vi "GUI_Tape_Alignment.vi"() -> ()   [LabVIEW 2020]
uses:
  Shared/GUI_Template/GUI_master/tcp_new_data_event.ctl
  Shared/GUI_Template/GUI_master/tcp new data cluster.ctl
  <vilib>/addons/_JKI.lib/Network_Streams_Connection.llb/NetworkCommand--Cluster.ctl
  <vilib>/addons/_JKI.lib/Network_Streams_Connection.llb/PublicSettings.ctl
  <vilib>/addons/_JKI.lib/Network_Streams_Connection.llb/NetworkConnection.lvclass/NetworkConnection.ctl
  <vilib>/Analysis/NI_AALPro.lvlib
  <vilib>/addons/_JKI.lib/Network_Streams_Connection.llb/NetworkConnection.lvclass
panel:
  in  "Check beam quality":bool
  in  "Zpos Scan":bool
  in  "2ndmomW0y::1":dbl caption="w0 Y" min=0.0 max=999999.0
  in  "MaxCounts::1":dbl caption="Max Counts" min=0.0 max=999999999.0
  in  "xyzuvw::2":string caption="Hex position"
  out "slow response":string
  in  "?":T1(tab)
  out "Zpos and w0 Y":dbl(graph)
  out "Alignment attempts":i32
  out "Waveform Chart 2":u32(graph)
  out "Movement time":u32
  out "Alignment time":u32
  out "Waveform Chart 3":u32(graph)
  out "Waveform Chart 4":i32(graph)
  out "Waveform Chart":cluster{"centroidx::1":dbl, "centroidy::1":dbl}(graph)
  out "Zpos and w0 Y 2":dbl(graph)
  out "X Graph":T2(graph)
  out "Y Graph":T3(graph)
  out "X slope":dbl
  out "Y slope":dbl
  out "Y error":dbl
  out "X error":dbl
  in  "Calibration steps":dbl=8.0
  in  "Calibration Angle":cluster{"X":dbl, "Y":dbl}={"X"=0.01, "Y"=0.01}
  in  "Export":bool caption="Export calibration"
  in  "Import":bool caption="Import calibration"
  in  "Diagnostic type":enum16{"Max counts", "w0 Y"}(ring)
  in  "Disable Zpos Scan":bool
  in  "zpos scan increment":dbl=0.1
  in  "zpos scan range":dbl=2.0
  in  "w0 Y Cutoff":dbl=60.0
  in  "Buffer":dbl=0.9 format="%#_13g"
  in  "Accuracy limit":cluster{"X":dbl, "Y":dbl}={"X"=5.0, "Y"=5.0}
  in  "Disable pointing correction":bool
  in  "Max counts cutoff":dbl=2000.0
  out "Connected?":bool
  in  "Message To Send":T4={"Command"="Alignment Done!", "Arguments"=variant(string "Arguments are variants. Wire anything!"), " Msg Id"=0}
  in  "Settings":T5={"My Name"="AlignmentGUI", "Remote IP Address"="", "Remote Name"="TapeDrive"}
  out "Public Settings":T5
  out "Message count":i32
  out "Incoming Messages":T4[](array[typedef])
  in  "Target.Y::1":dbl caption="Target Y" min=0.0 max=2000.0
  in  "Target.X::1":dbl caption="Target X" min=0.0 max=2000.0
  in  "Stop":bool
  out "Remaining States":string
  out "Current State":string
  in  "Calibrate":bool
  in  "wangle::2":dbl caption="W" min=-10.0 max=10.0 step=0.01 format="%.5f"
  in  "vangle::2":dbl caption="V" min=-5.0 max=5.0 step=0.01 format="%.5f"
  in  "centroidy::1":dbl caption="Centroid Y" min=0.0 max=0.0
  in  "centroidx::1":dbl caption="Centroid X" min=0.0 max=0.0
  in  "ypos::2":dbl caption="Y" min=-25.0 max=25.0 step=0.01 format="%.5f"
  in  "xpos::2":dbl caption="X" min=-25.0 max=25.0 step=0.01 format="%.5f"
  in  "zpos::2":dbl caption="Z" min=-25.0 max=25.0 step=0.01 format="%.5f"
  in  "uangle::2":dbl caption="U" min=-5.0 max=5.0 step=0.01 format="%.5f"
  out "tcp data event":T6
  out "error IO 2":errorcluster
  in  "GUIdevice 2":string="HEX-PL1-2"
  in  "GUIdevice 1":string="CAM-PL1-SideSpec"
  in  "Align Tape":bool
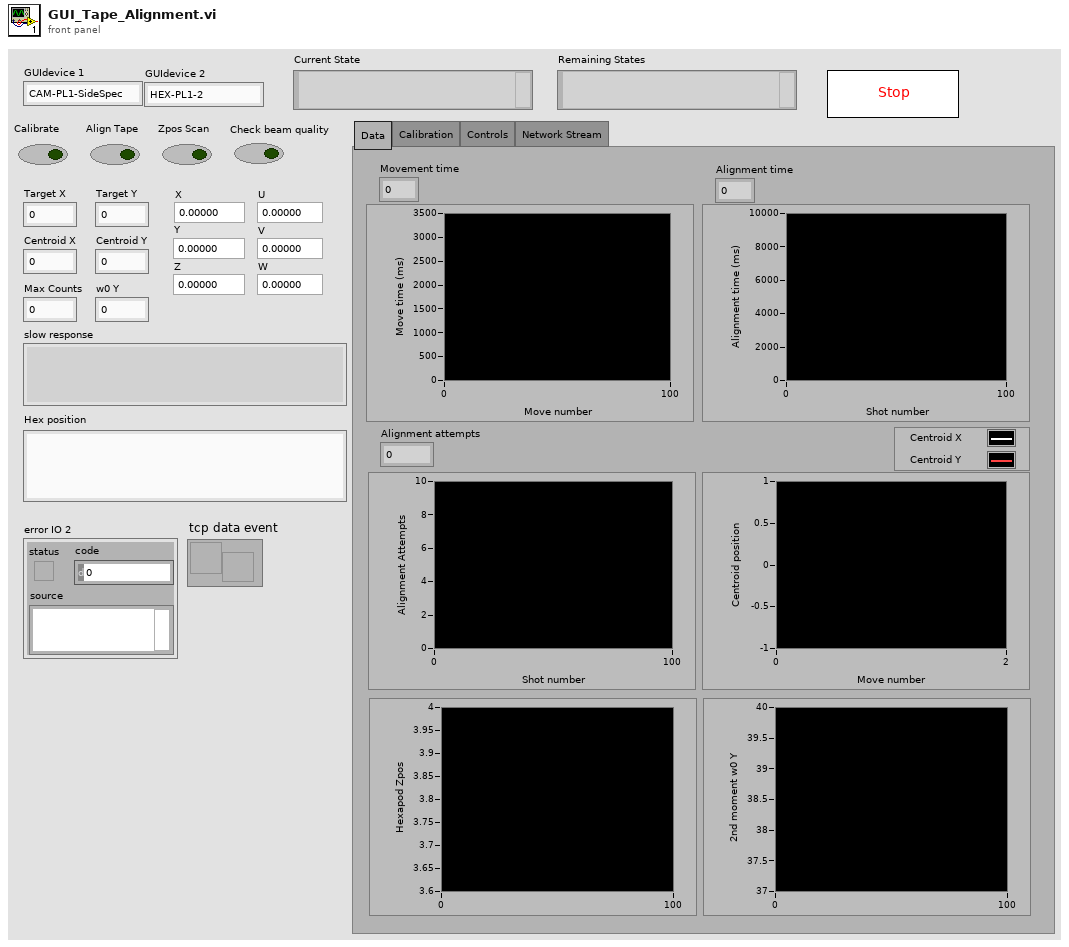
[diagram p1: front panel]
types:
  T1 = enum32{"Data", "Calibration", "Controls", "Network Stream"}
  T2 = cluster{"Centroids.x":dbl[], "Best Linear Fit":dbl[]}[]
  T3 = cluster{"Centroids.y":dbl[], "Best Linear Fit":dbl[]}[]
  T4 = typedef "NetworkConnection.lvclass/NetworkCommand--Cluster.ctl" = cluster{"Command":string, "Arguments":variant, " Msg Id":i32}
  T5 = typedef "NetworkConnection.lvclass/PublicSettings.ctl" = cluster{"My Name":string, "Remote IP Address":string, "Remote Name":string}
  T6 = typedef "tcp_new_data_event.ctl" = refnum<user-event>
  T7 = typedef "tcp new data cluster.ctl" = cluster{"EventEnum":enum16{"new data", "connection status update"}, "Device name":string}
  T8 = enum32{"Invalid", "Standard", "Closed", "Hidden", "Minimized", "Maximized"}
  T9 = enum32{"invalid app kind", "Development System", "Run Time System", "Student Edition", "Embedded LabVIEW", "Evaluation", "Custom"}
  T10 = cluster{"Messages[0]":T4, "Messages[1]":T4, "Messages[2]":T4, "Messages[3]":T4, "Messages[4]":T4, "Messages[5]":T4, "Messages[6]":T4, "Messages[7]":T4, "Messages[8]":T4}
  T11 = cluster{"Core":cluster{"Current VI Reference":refnum<vi>, "Close Panel on Exit?":bool}, "Difference":cluster{"X":dbl, "Y":dbl}, "Scale Factor":cluster{"X":dbl, "Y":dbl}, "Centroids":cluster{"Centroids.x":dbl[], "Centroids.y":dbl[]}, "Calibration Angle ":cluster{"X":dbl, "Y":dbl}, "Accuracy limit":cluster{"X":dbl, "Y":dbl}, "Calibration steps":dbl, "NetworkConnection out":refnum<class "NetworkConnection.lvclass">, "Messages":i32, "Alignment attempts":i32, "Timer":cluster{"T1":i32, "T2":i32}, "Hexapod positions":cluster{"P1":string, "P2":string}, "Beam diagnostic cutoffs":cluster{"MaxCounts":dbl, "w0 Y":dbl}, "Hexapod zscan data":cluster{"Hexapod zscan positions":dbl[], "Hexapod zscan diagnostic":dbl[], "Index":i32, "Best Zpos":dbl}, "Diagnostic type":string}
  T12 = cluster{"Hexapod zscan positions":dbl[], "Hexapod zscan diagnostic":dbl[], "Index":i32, "Best Zpos":dbl}
  T13 = cluster{"Centroids.x":dbl[], "Centroids.y":dbl[]}
  T14 = cluster{"Current VI Reference":refnum<vi>, "Close Panel on Exit?":bool}
  T15 = cluster{"Centroids.x":dbl[], "Best Linear Fit":dbl[]}
  T16 = cluster{"Centroids.y":dbl[], "Best Linear Fit":dbl[]}
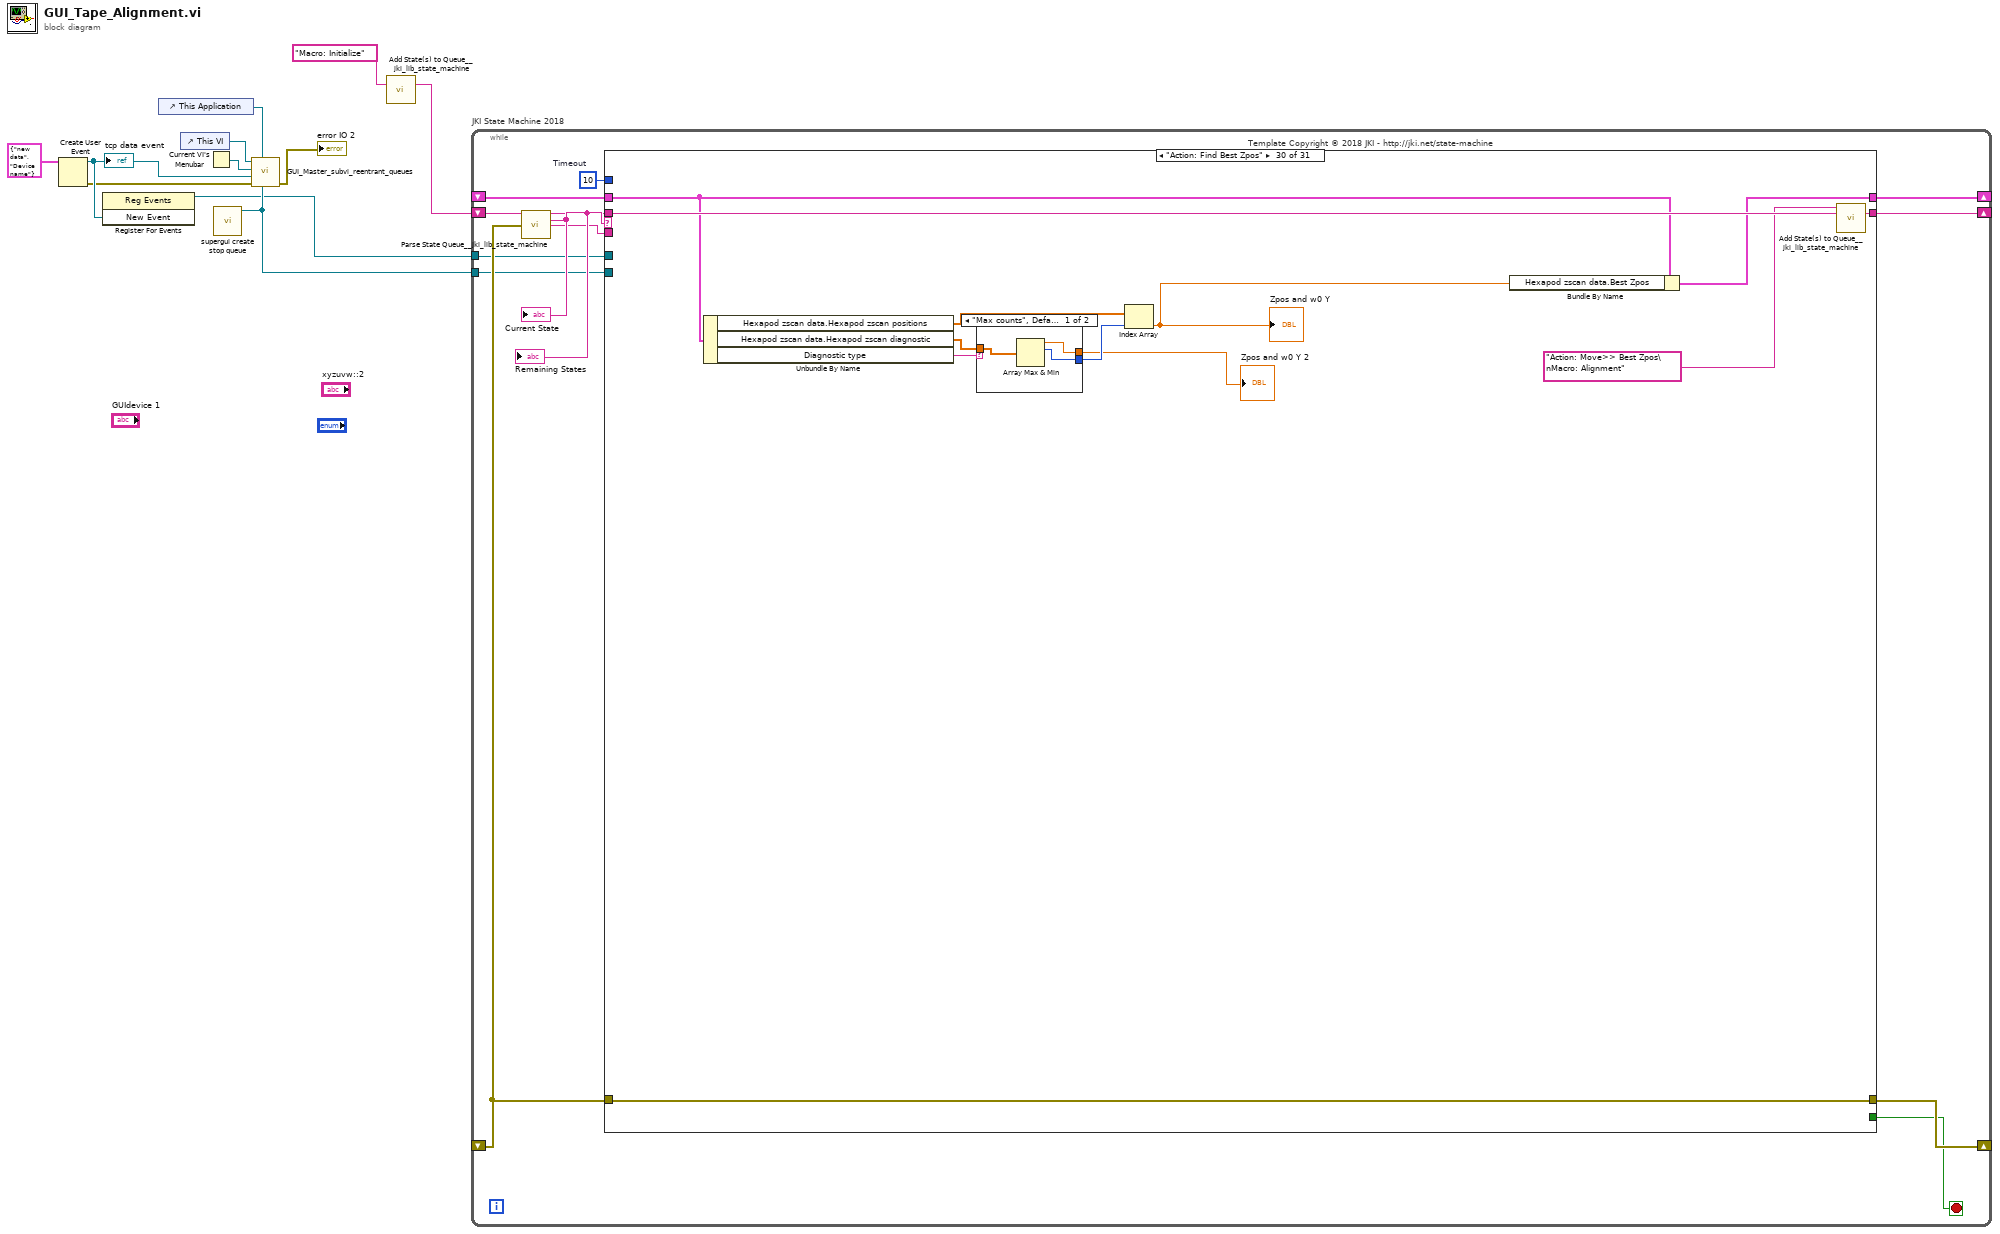
[diagram p0: block diagram]
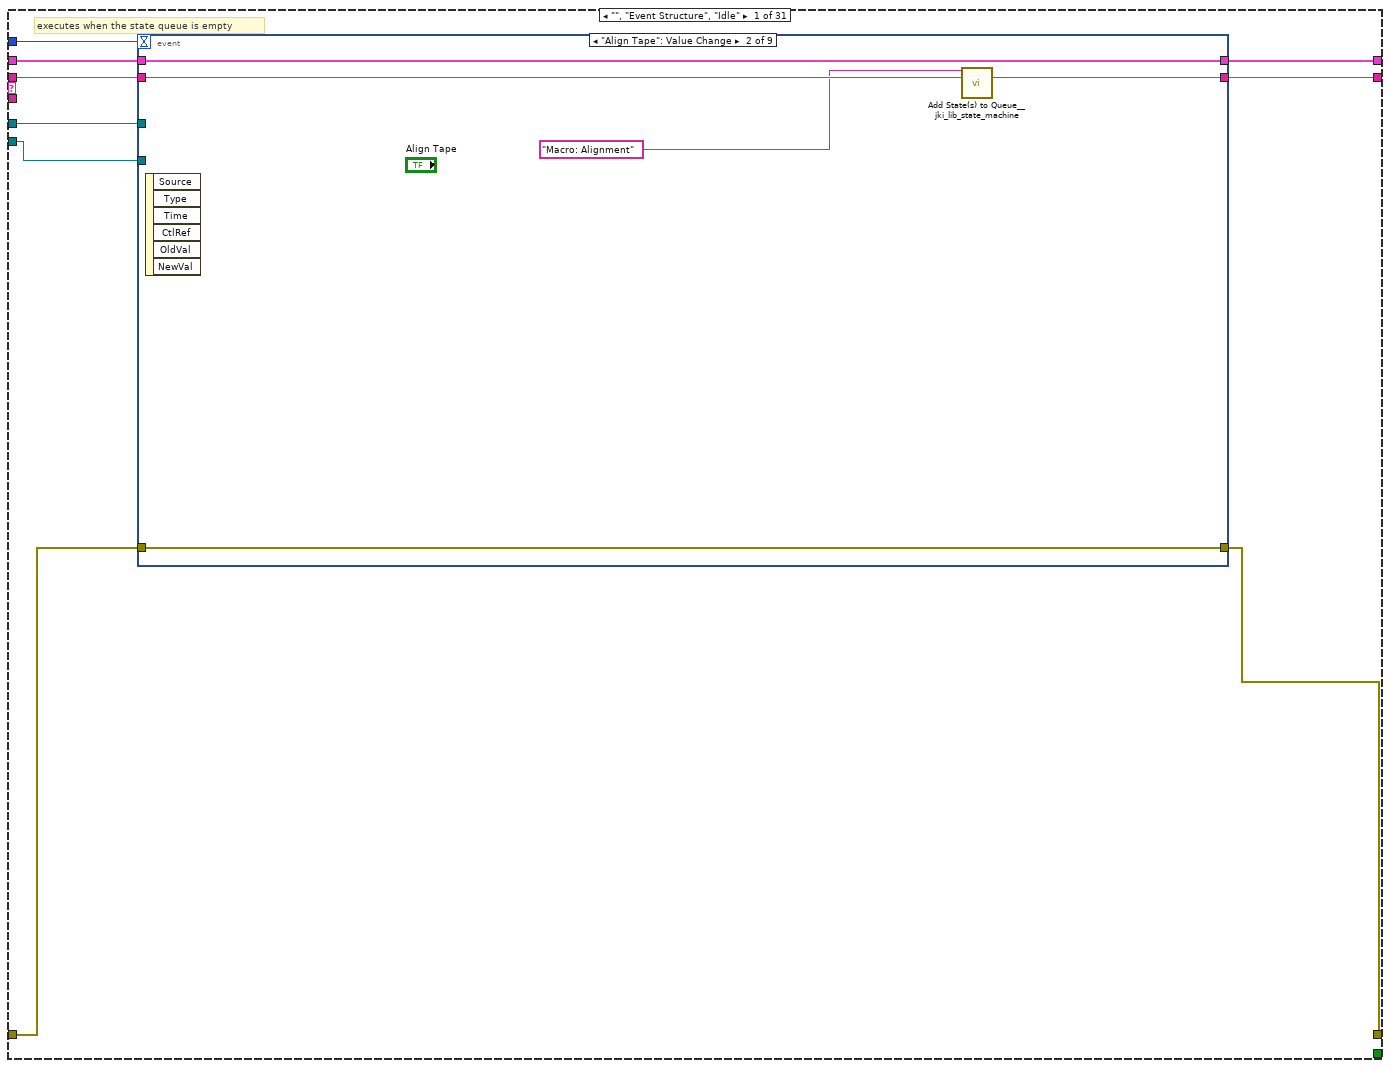
[diagram p2: hidden frame]
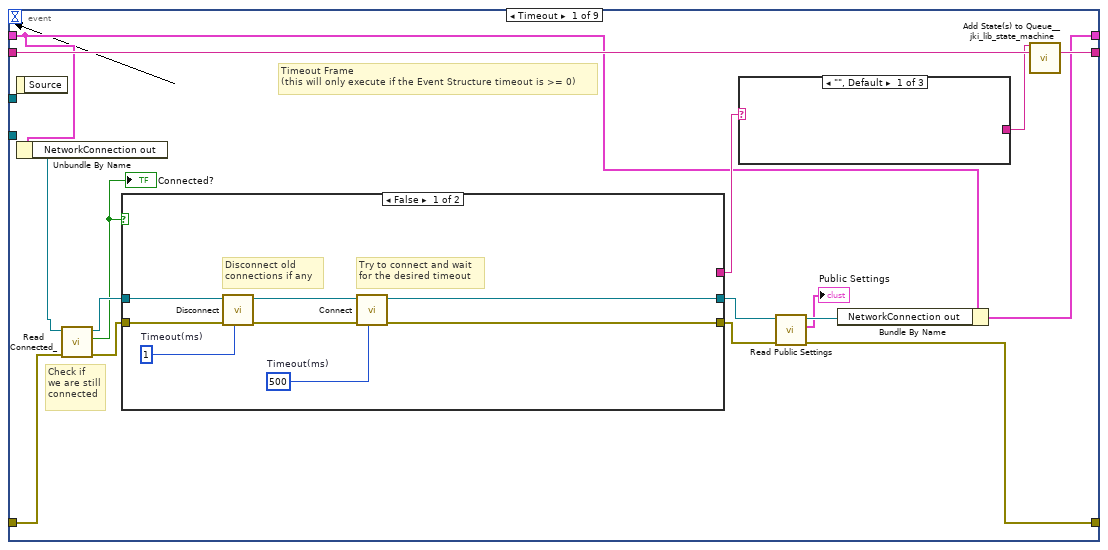
[diagram p3: hidden frame]
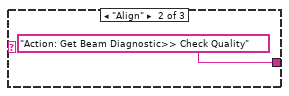
[diagram p4: hidden frame]
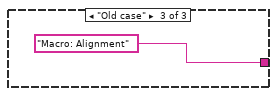
[diagram p5: hidden frame]
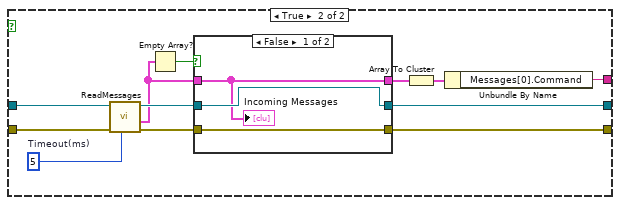
[diagram p6: hidden frame]
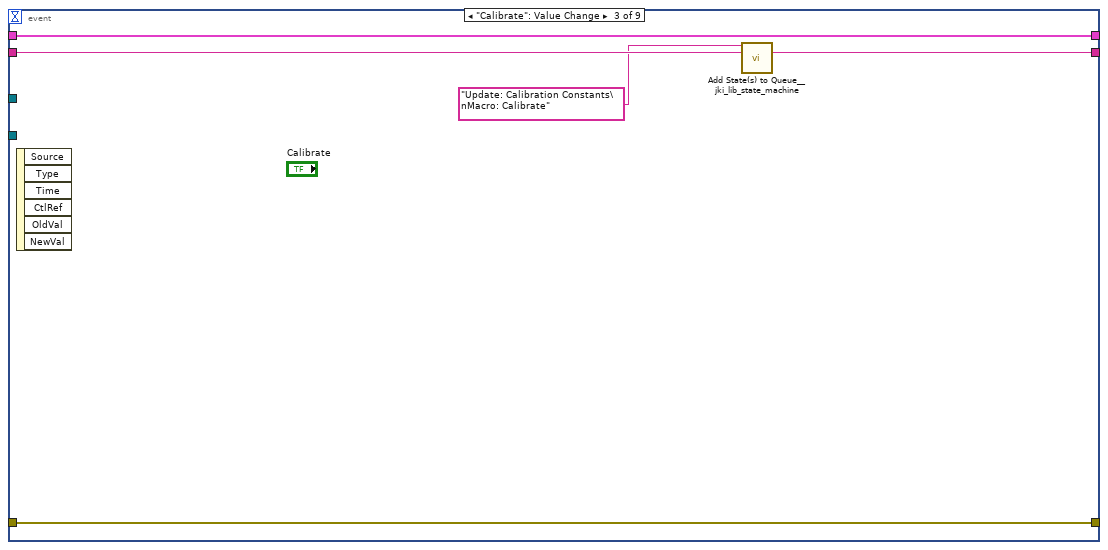
[diagram p8: hidden frame]
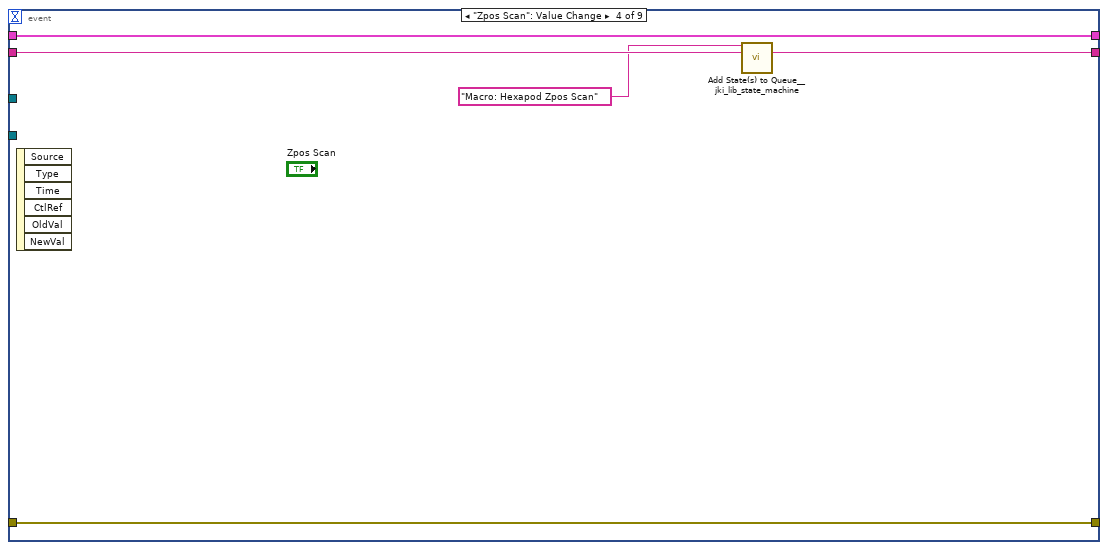
[diagram p9: hidden frame]
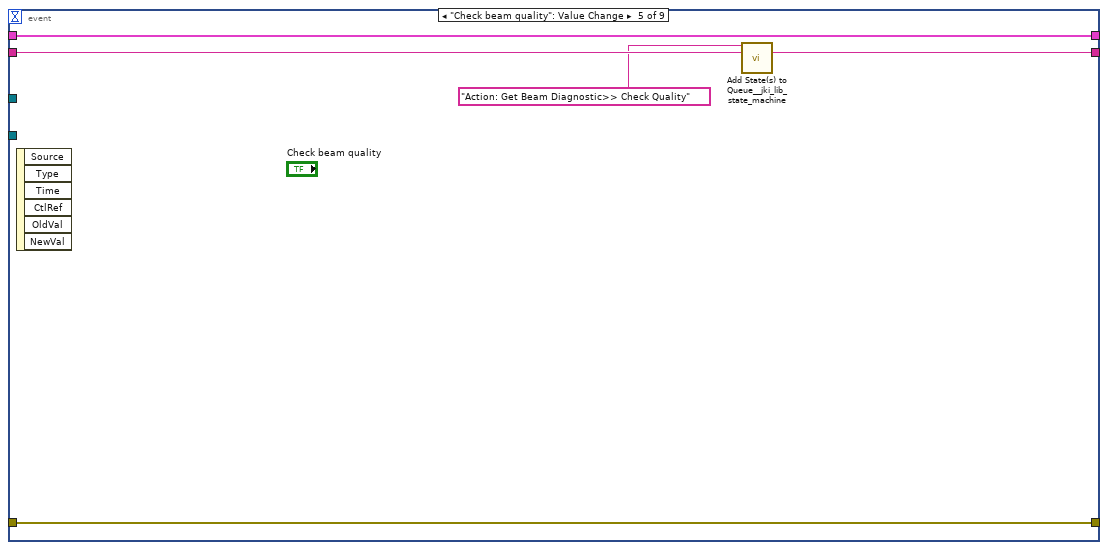
[diagram p10: hidden frame]
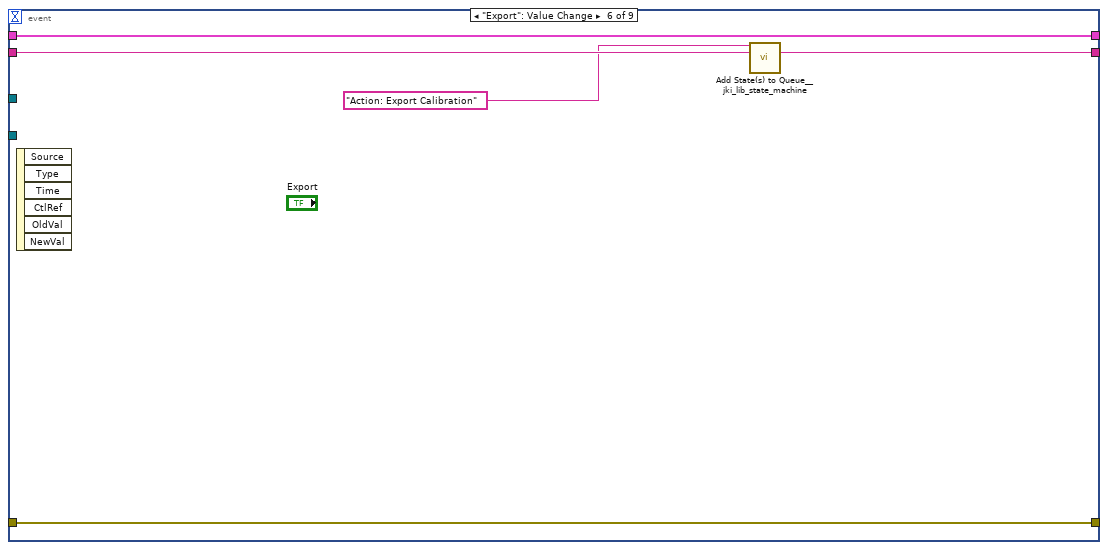
[diagram p11: hidden frame]
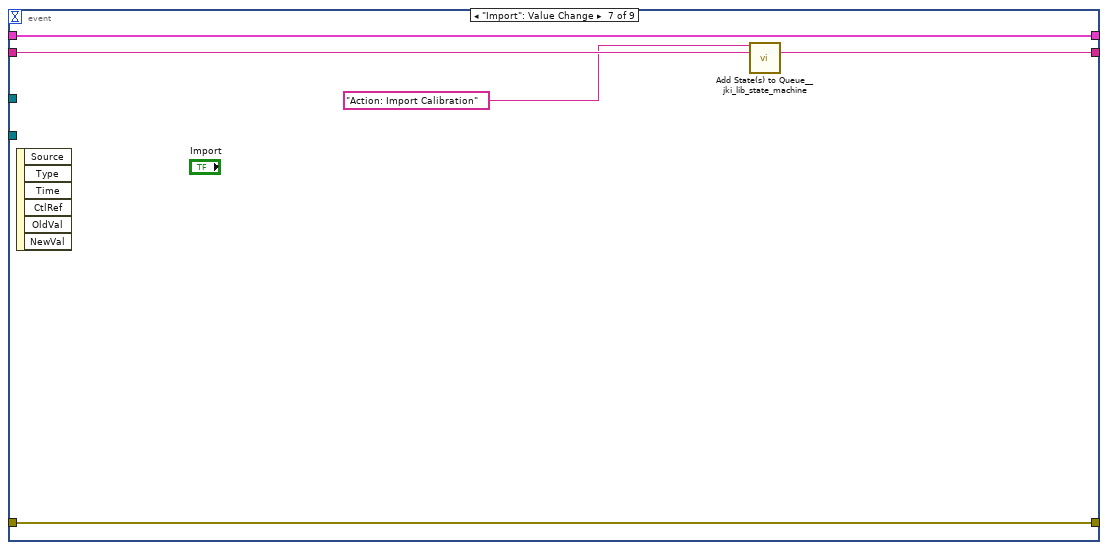
[diagram p12: hidden frame]
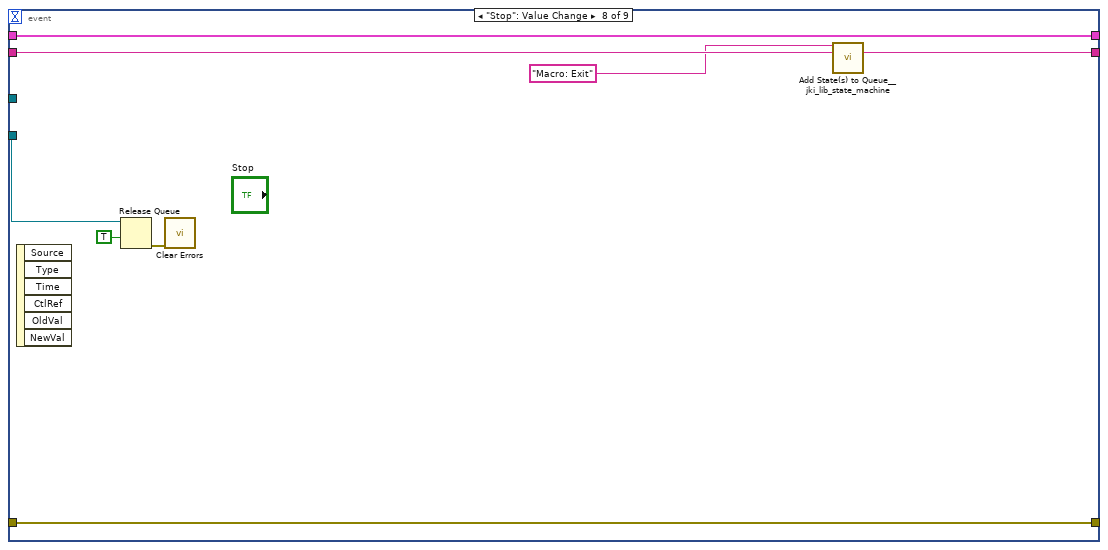
[diagram p13: hidden frame]
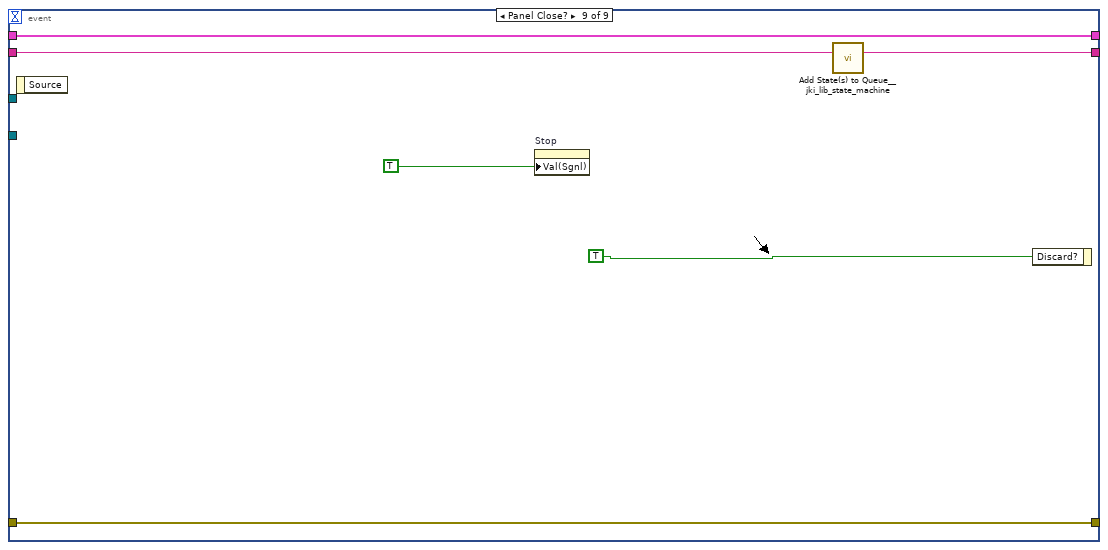
[diagram p14: hidden frame]
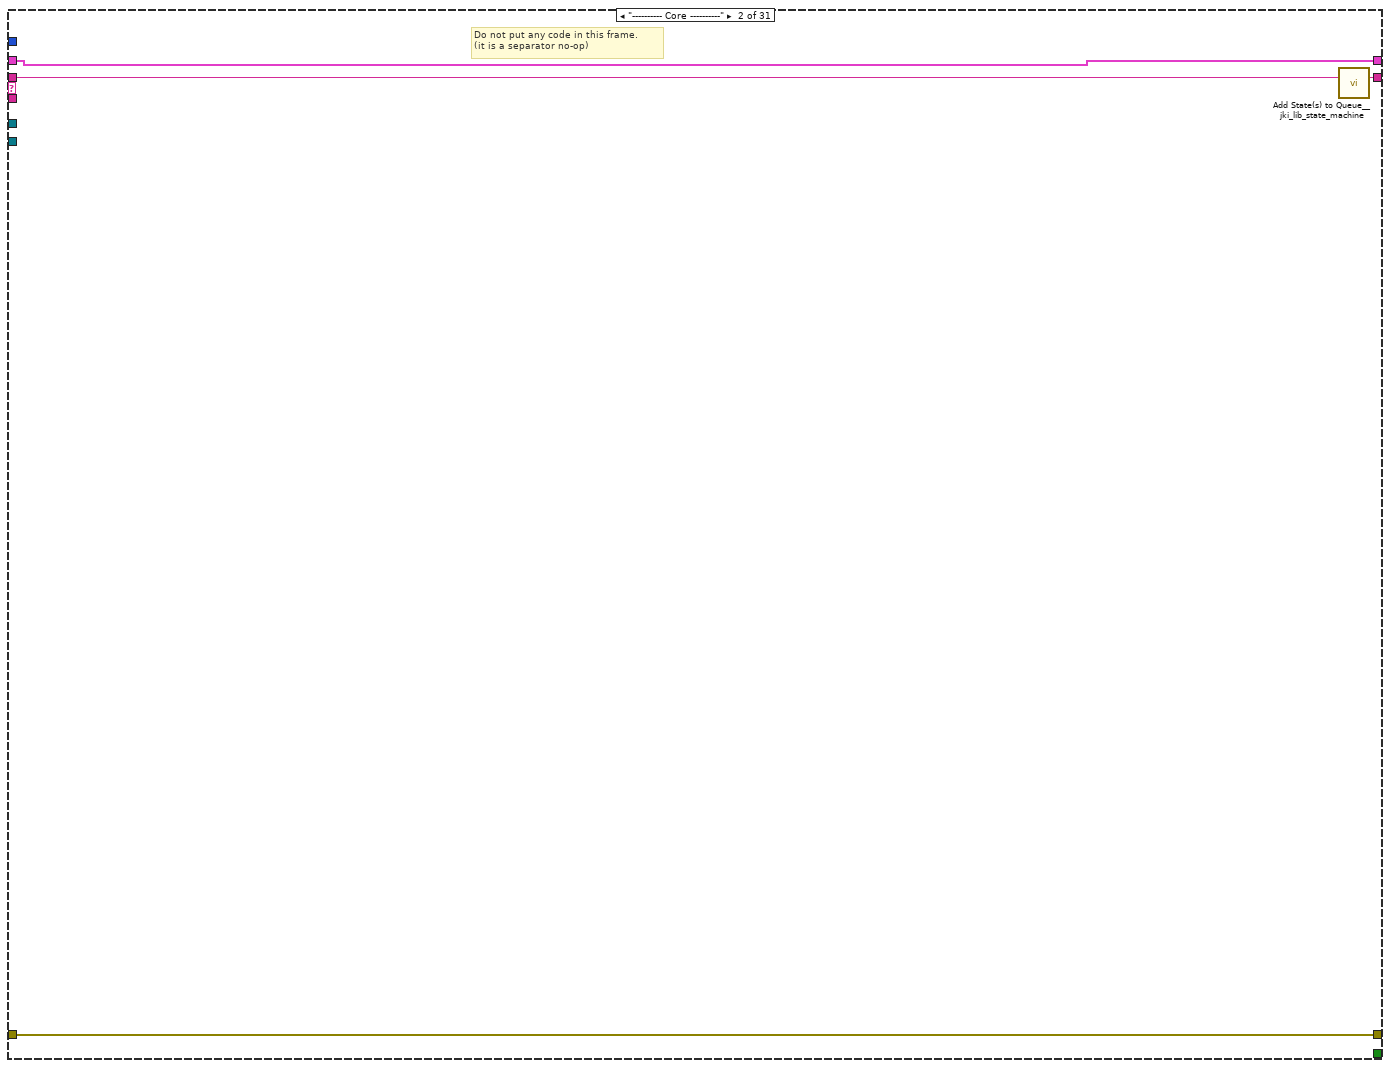
[diagram p15: hidden frame]
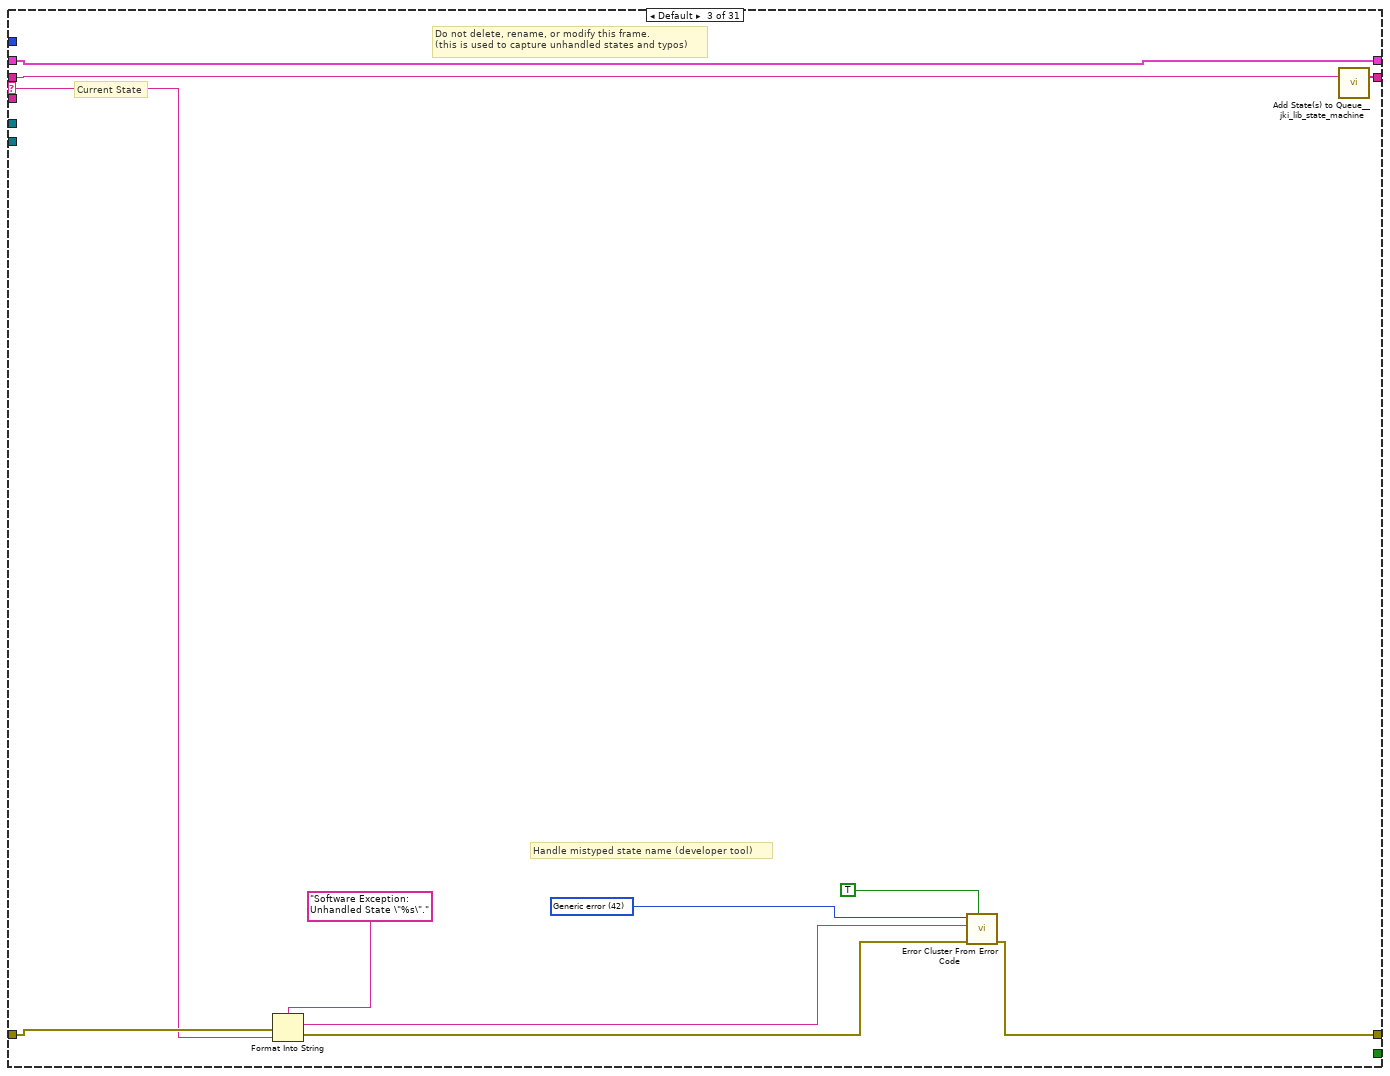
[diagram p16: hidden frame]
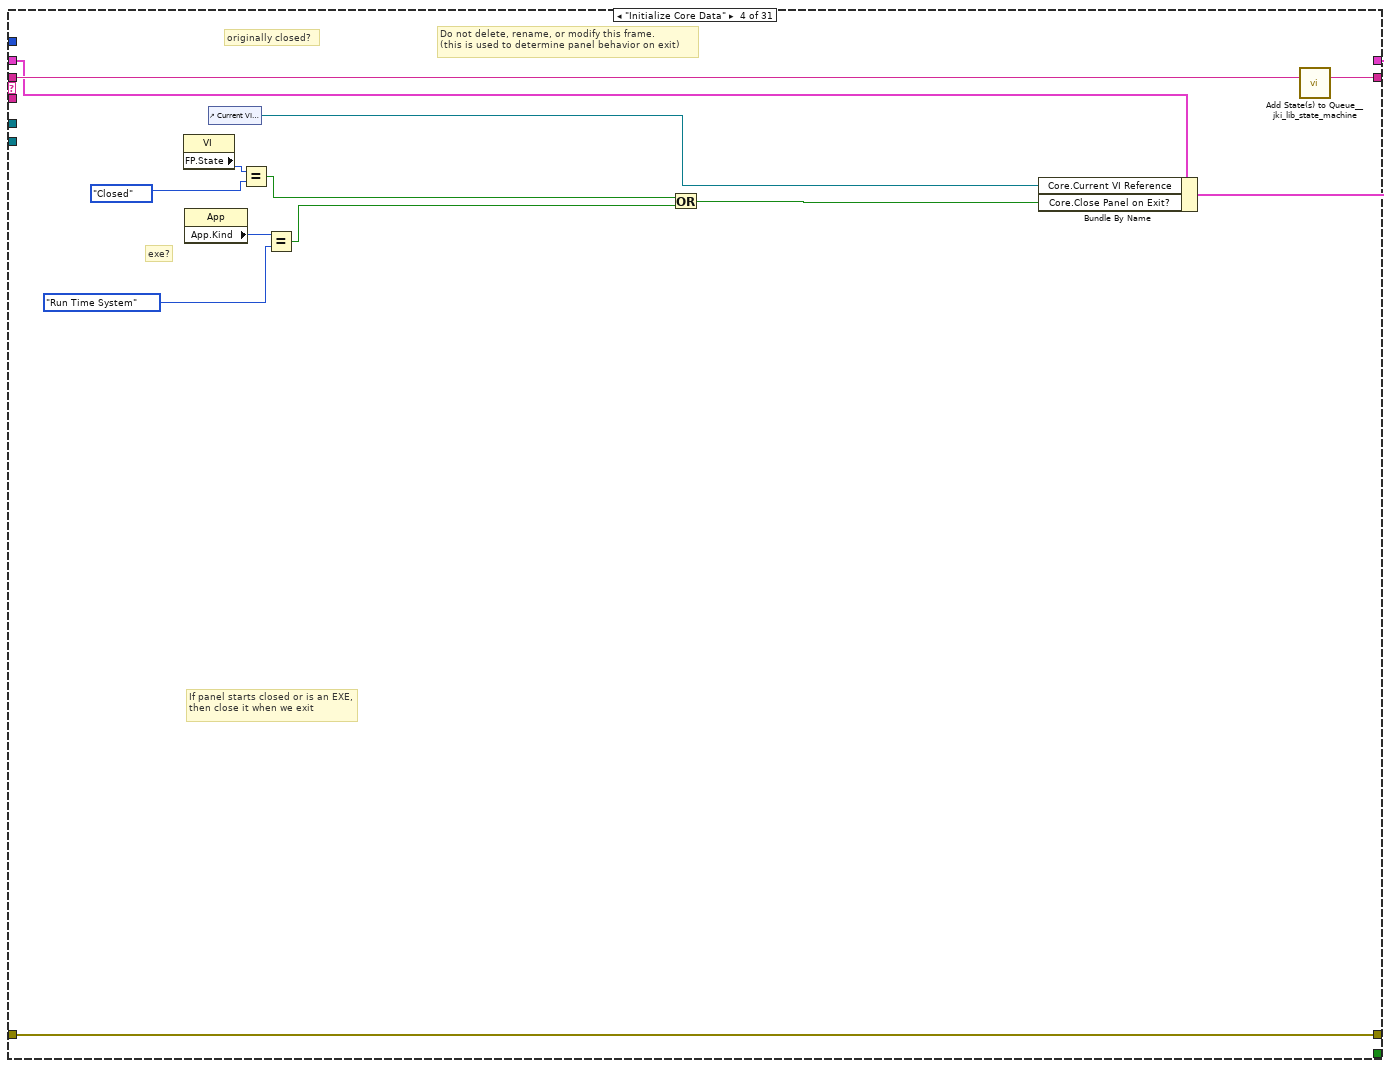
[diagram p17: hidden frame]
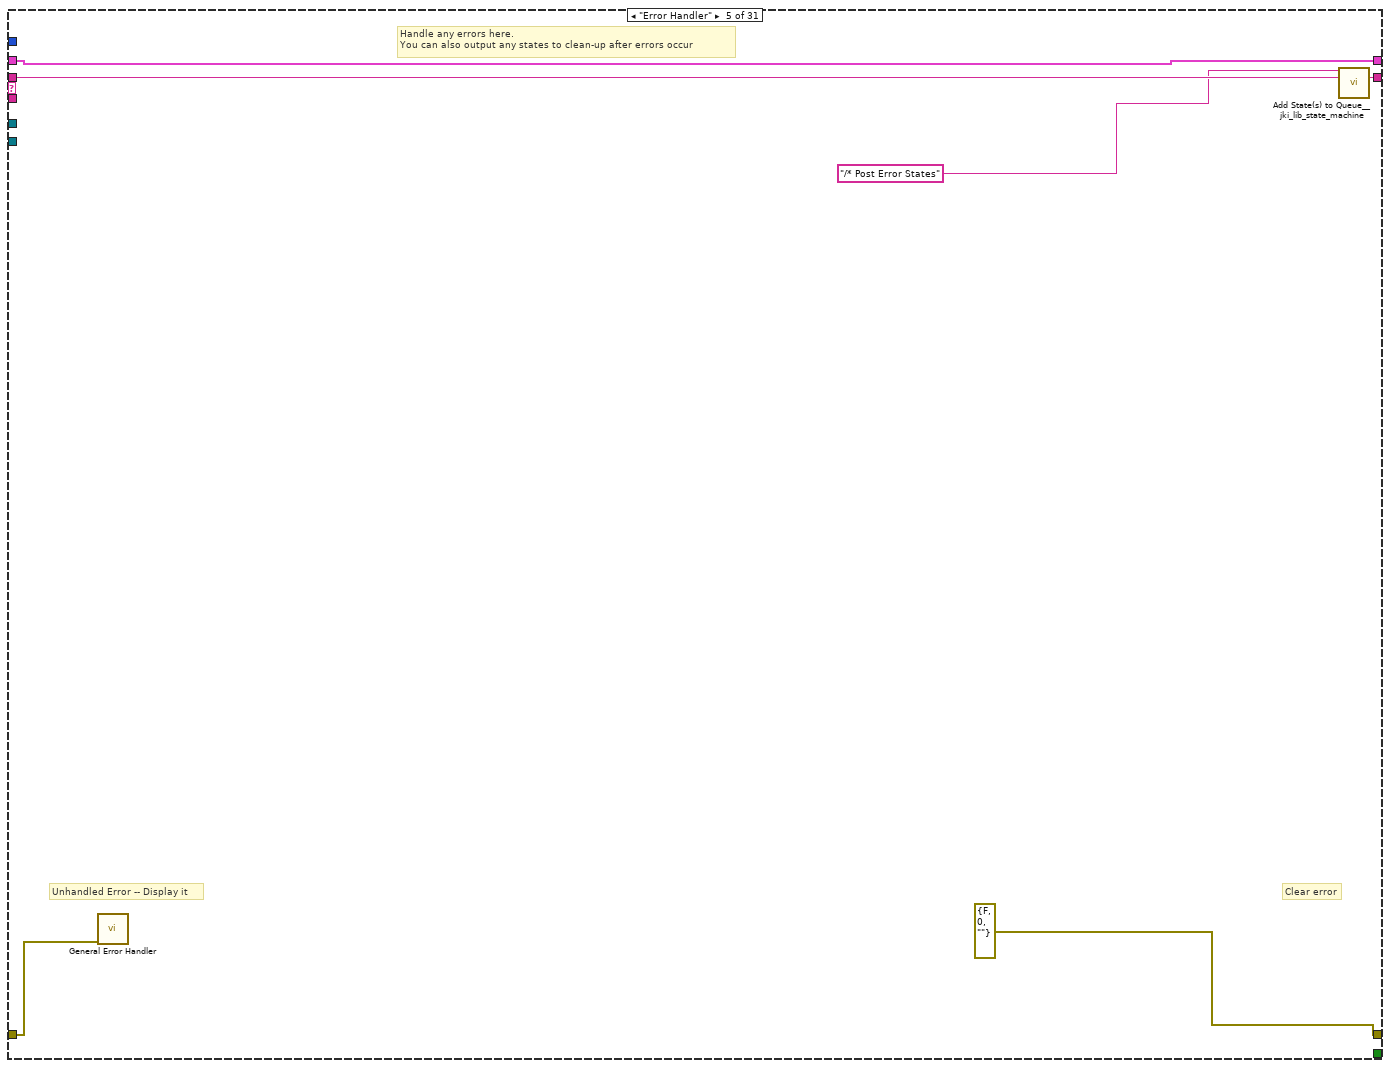
[diagram p18: hidden frame]
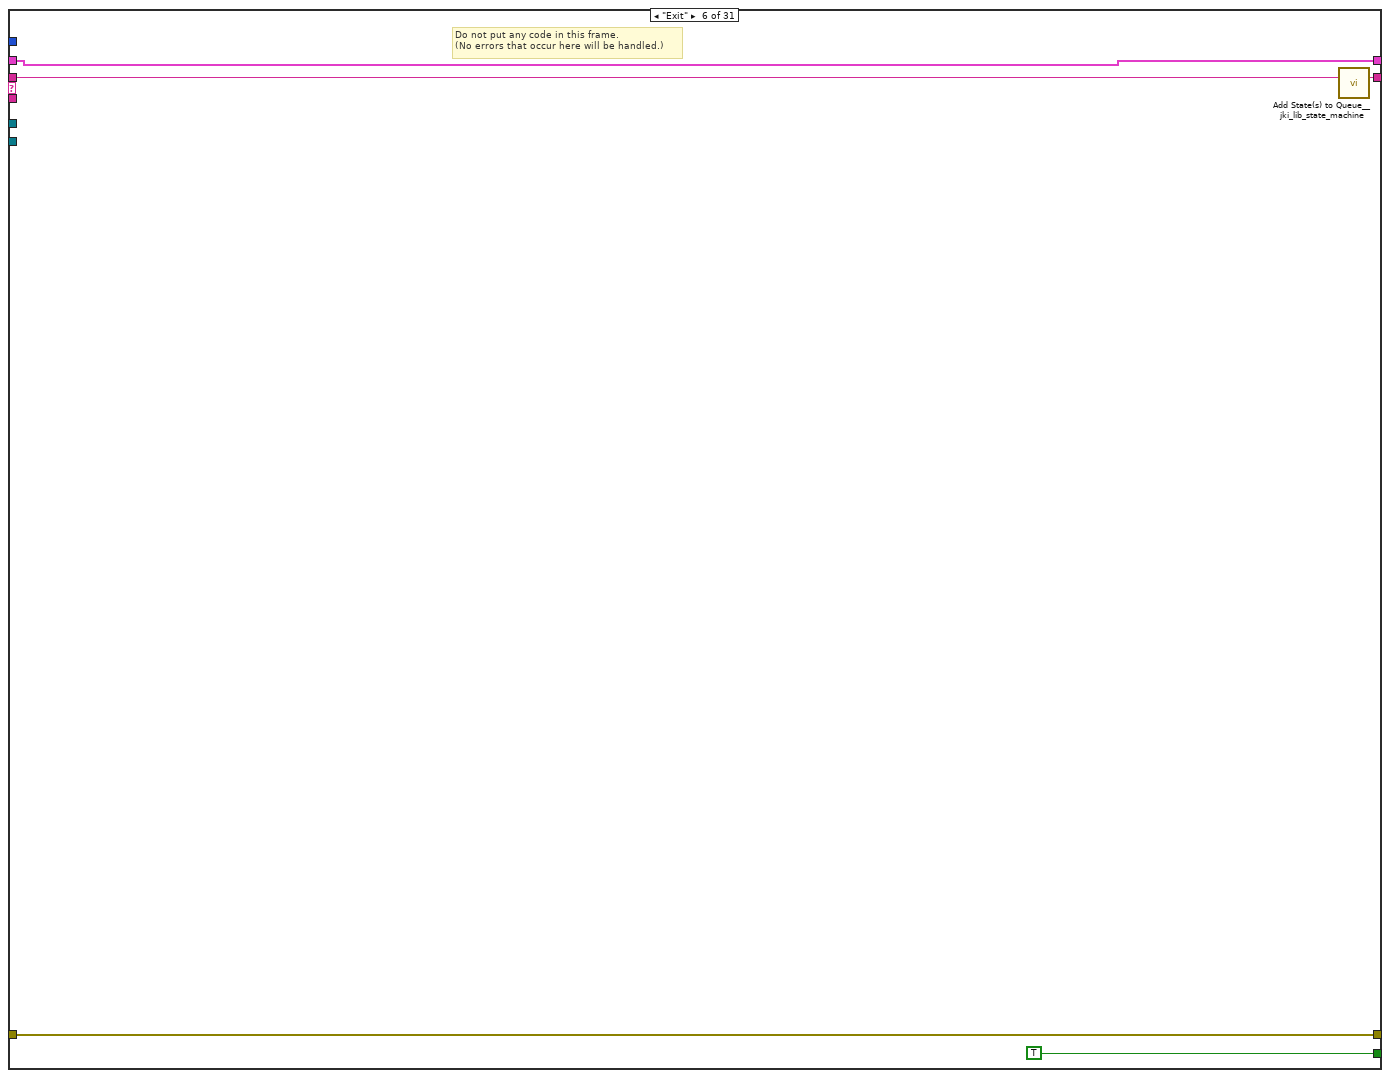
[diagram p19: hidden frame]
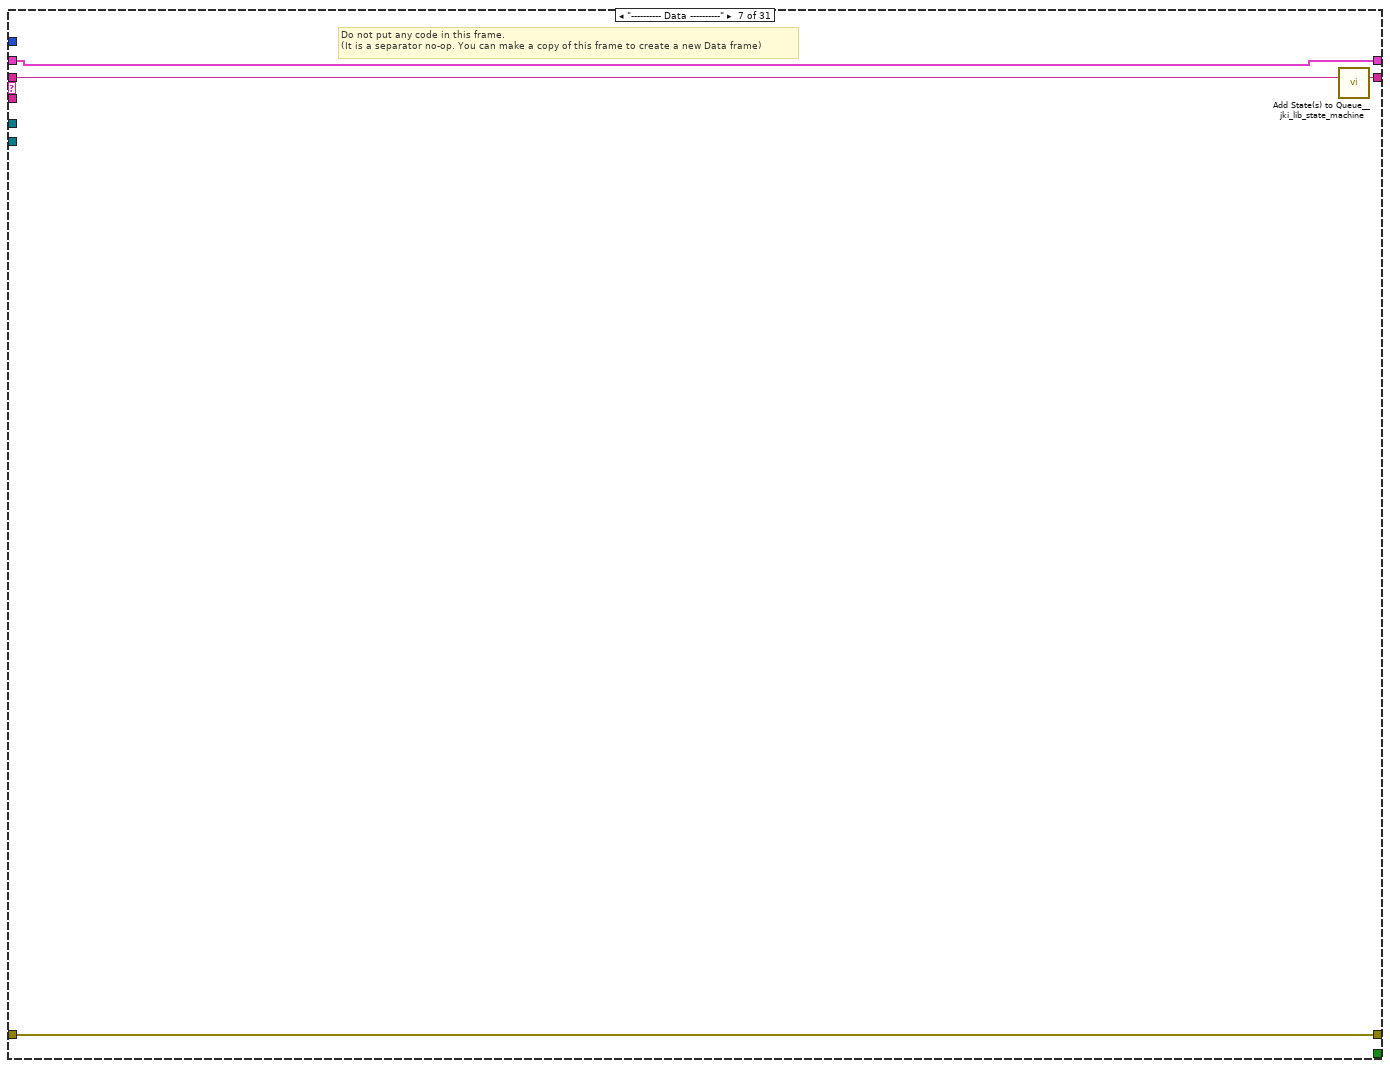
[diagram p20: hidden frame]
diagram:
  n1 = Create User Event(user event datatype=T7 {"EventEnum"=enum."new data", "Device name"="Device name"} ("New Event")) -> (user event=w8:refnum<user-event>, error out=w7:errorcluster)  [unwired: 1 in]
  "tcp data event" <- w8
  n2 = register-events(w8) -> (reference out=w1:refnum<event-registration>)  [unwired: 2 in, 1 out]
  n3 = control-ref of="This Application"() -> (w9:refnum<vi>)
  n4 = control-ref of="This VI"() -> (w4:refnum<vi>)
  n5 = Current VI's Menubar() -> (w5:refnum<k9>)
  n6 = call "supergui create stop queue.vi"() -> ("STOP Queue out"=w2:refnum<queue>)  [unwired: 11 in]
  n7 = call "GUI_Master_subvi_reentrant_queues.vi"("STOP Queue in"=w2, "This Application"=w9, "error in (no error)"=w7, "tcp data event"=w8, "Caller menu reference"=w5, "Caller VI ref"=w4) -> ("error out"=→"error IO 2":errorcluster)  [unwired: 5 in]
  n8 = call <vilib>:"Add State(s) to Queue__jki_lib_state_machine.vi"("State(s) in (\"\")"="Macro: Initialize") -> ("States Out"=w11:string)  [unwired: 14 in]
  n9 = while "JKI State Machine 2018" {
    shift-right: [w18] -> _
    shift-left: _ -> [w17]
    shift-right: [w20] -> _
    shift-left: _ -> [w15]
    shift-right: [w19] -> _
    shift-left: w11 -> [w21]
    tunnel: w1 -> [w14]
    tunnel: w2 -> [w13]
    stop <- w12 stop-if-true
    w16 = 10  # Timeout
    # "Template Copyright © 2018 JKI - http://jki.net/state-machine"
    n10 = call <vilib>:"Parse State Queue__jki_lib_state_machine.vi"("State Queue"=w21, "Error In (no error)"=w15) -> ("Remaining States"=w23:string, "Current State"=w24:string, "Arguments"=w22:string)  [unwired: 11 in]
    "Current State" <- w24
    "Remaining States" <- w23
    n11 = case shown="\"Action: Find Best Zpos\"" w24 {
      selector: w24 -> [_ _ w126 _ _ _ _ _ _ _ _ _ _ _ _ _ _ _ _ _ _ _ _ _ _ _ _ _ _ _ _]
      tunnel: w23 -> [w33 w125 w130 w149 w155 w160 w164 w184 w192 w196 w200 w206 w217 w286 w291 w301 w313 w340 w352 w359 w365 w373 w378 w390 w426 w558 w566 w577 w588 w627 w651]
      tunnel: w22 -> [_ _ _ _ _ _ _ _ _ _ _ w201 w211 _ _ _ _ _ _ _ _ _ _ w388 w447 _ _ _ w586 _ _]
      tunnel: w17 -> [w31 w122 w128 w142 w152 w158 w161 _ w188 w193 w198 w204 w213 w283 w288 w294 w317 w336 w349 w356 w363 w372 w375 w387 w446 w554 w564 w572 w579 w624 w644]
      tunnel: [w30 w123 w132 w146 errorcluster {"status"=FALSE, "code"=0, "source"=""} ("error out") w157 w162 w181 w185 w194 w197 w202 w214 w284 w289 w303 w328 w341 w350 w357 w366 w368 w376 w380 w439 w556 w560 w567 w581 w625 w638] -> w20
      tunnel: w15 -> [w29 w123 w131 w146 w151 w157 w162 w181 w189 w194 w197 w203 w215 w284 w289 w303 w328 w341 w350 w357 w366 w368 w376 w379 w445 w556 w561 w568 w582 w625 w648]
      tunnel: [w32 w124 w129 w148 w154 w159 w163 w183 w191 w195 w199 w205 w216 w285 w290 w304 w329 w342 w351 w358 w367 w374 w377 w389 w448 w557 w565 w576 w587 w626 w650] -> w19
      tunnel: [_ _ _ _ _ TRUE _ _ _ _ _ _ _ _ _ _ _ _ _ _ _ _ _ _ _ _ _ _ _ _ _] -> w12
      tunnel: [w28 w122 w128 w147 w152 w158 w161 w182 w188 w193 w198 w204 w213 w283 w288 w292 w316 w337 w349 w356 w362 w371 w375 w386 w424 w555 w564 w575 w583 w623 w645] -> w18
      tunnel: w16 -> [w27 _ _ _ _ _ _ _ _ _ _ _ _ _ _ _ _ _ _ _ _ _ _ _ _ _ _ _ _ _ _]
      tunnel: w14 -> [w26 _ _ _ _ _ _ _ _ _ _ _ _ _ _ _ _ _ _ _ _ _ _ _ _ _ _ _ _ _ _]
      tunnel: w13 -> [w25 _ _ _ _ _ _ _ _ _ _ _ _ _ _ _ _ _ _ _ _ _ _ _ _ _ _ _ _ _ _]
      frame "", "Event Structure", "Idle" {
        # "executes when the state queue is empty"
        n12 = event shown="[1] \"Align Tape\": Value Change" {
          selector: _ -> [_ _ _ _ _ _ _ _ _]
          dyn-events: _ -> [_ _ _ _ _ _ _ _ _]
          timeout: w27 -> [_ _ _ _ _ _ _ _ _]
          tunnel: w33 -> [w49 w82 w86 w91 w96 w100 w105 w115 w121]
          tunnel: [w48 w81 w84 w89 w94 w101 w106 w114 w120] -> w32
          tunnel: w31 -> [w39 w78 w87 w92 w97 w102 w107 w112 w118]
          tunnel: [w36 w80 w83 w88 w93 w98 w103 w113 w119] -> w30
          tunnel: w29 -> [w44 w80 w83 w88 w93 w98 w103 w113 w119]
          tunnel: [w40 w78 w87 w92 w97 w102 w107 w112 w118] -> w28
          tunnel: w26 -> [_ _ _ _ _ _ _ _ _]
          tunnel: w25 -> [_ _ _ _ _ _ _ w108 _]
          event Timeout {
            # "Check if\nwe are still\nconnected"
            # "Timeout Frame\n(this will only execute if the Event Structure timeout is >= 0)"
            n13 = event-data() -> ()  [unwired: 1 in, 1 out]
            n14 = Unbundle By Name(w39) -> ("NetworkConnection out"=w41:refnum<class "NetworkConnection.lvclass">)
            n15 = call <vilib>:"Read Connected_.vi"("error in (no error)"=w44, "NetworkConnection in"=w41) -> ("error out"=w47:errorcluster, "Connected?"=w45:bool, "NetworkConnection out"=w46:refnum<class "NetworkConnection.lvclass">)  [unwired: 7 in]
            "Connected?" <- w45
            n16 = case shown="False" w45 {
              tunnel: w47 -> [w55 w69]
              tunnel: w46 -> [w57 w70]
              tunnel: [w58 w64] -> w38
              tunnel: [w59 w63] -> w37
              tunnel: [_ w67] -> w43
              frame False {
                w52 = 500  # Timeout(ms)
                w53 = 1  # Timeout(ms)
                # "Try to connect and wait\nfor the desired timeout"
                # "Disconnect old\nconnections if any"
                n17 = call <vilib>:"Disconnect.vi"("Timeout ms (1000)"=w53, "error in (no error)"=w55, "NetworkConnection in"=w57) -> ("error out"=w54:errorcluster, "NetworkConnection out"=w56:refnum<class "NetworkConnection.lvclass">)  [unwired: 7 in]
                n18 = call <vilib>:"Connect.vi"("Timeout(ms)"=w52, "error in (no error)"=w54, "NetworkConnection in"=w56) -> ("error out"=w59:errorcluster, "NetworkConnection out"=w58:refnum<class "NetworkConnection.lvclass">)  [unwired: 6 in, 1 out]
              }
              frame True {
                w71 = 5  # Timeout(ms)
                n19 = call <vilib>:"ReadMessages.vi"("Timeout(ms)"=w71, "error in (no error)"=w69, "NetworkConnection in"=w70) -> ("error out"=w62:errorcluster, "Messages"=w60:T4[], "NetworkConnection out"=w65:refnum<class "NetworkConnection.lvclass">)  [unwired: 4 in, 2 out]
                n20 = Empty Array?(array=w60) -> (empty?=w66:bool)
                n21 = case shown="False" w66 {
                  tunnel: w65 -> [w74 w77]
                  tunnel: [w74 w77] -> w64
                  tunnel: [w73 w76] -> w63
                  tunnel: w62 -> [w73 w76]
                  tunnel: [w72 w75] -> w61
                  tunnel: w60 -> [w72 w75]
                  frame False {
                    "Incoming Messages" <- w72
                  }
                  frame True {
                  }
                }
                n22 = Array To Cluster(array=w61) -> (cluster=w68:T10)
                n23 = Unbundle By Name(w68) -> ("Messages[0].Command"=w67:string)
              }
            }
            n24 = case shown="\"\", Default" w43 {
              tunnel: [_ "Action: Get Beam Diagnostic>> Check Quality" "Macro: Alignment"] -> w42
              frame "", Default {
              }
              frame "Align" {
              }
              frame "Old case" {
              }
            }
            n25 = call <vilib>:"Read Public Settings.vi"("error in (no error)"=w37, "NetworkConnection in"=w38) -> ("error out"=w36:errorcluster, "Public Settings"=→"Public Settings":T5, "NetworkConnection out"=w35:refnum<class "NetworkConnection.lvclass">)  [unwired: 7 in]
            n26 = Bundle By Name(cluster=w39, "NetworkConnection out"=w35) -> (w40:T11)
            n27 = call <vilib>:"Add State(s) to Queue__jki_lib_state_machine.vi"("State(s) in Front (\"\")"=w42, "State(s) in (\"\")"=w49) -> ("States Out"=w48:string)  [unwired: 13 in]
          }
          event "Align Tape": Value Change {
            n28 = event-data() -> ()  [unwired: 1 in, 6 out]
            n29 = call <vilib>:"Add State(s) to Queue__jki_lib_state_machine.vi"("State(s) in Front (\"\")"="Macro: Alignment", "State(s) in (\"\")"=w82) -> ("States Out"=w81:string)  [unwired: 13 in]
          }
          event "Calibrate": Value Change {
            n30 = event-data() -> ()  [unwired: 1 in, 6 out]
            n31 = call <vilib>:"Add State(s) to Queue__jki_lib_state_machine.vi"("State(s) in Front (\"\")"="Update: Calibration Constants\nMacro: Calibrate", "State(s) in (\"\")"=w86) -> ("States Out"=w84:string)  [unwired: 13 in]
          }
          event "Zpos Scan": Value Change {
            n32 = event-data() -> ()  [unwired: 1 in, 6 out]
            n33 = call <vilib>:"Add State(s) to Queue__jki_lib_state_machine.vi"("State(s) in Front (\"\")"="Macro: Hexapod Zpos Scan", "State(s) in (\"\")"=w91) -> ("States Out"=w89:string)  [unwired: 13 in]
          }
          event "Check beam quality": Value Change {
            n34 = event-data() -> ()  [unwired: 1 in, 6 out]
            n35 = call <vilib>:"Add State(s) to Queue__jki_lib_state_machine.vi"("State(s) in Front (\"\")"="Action: Get Beam Diagnostic>> Check Quality", "State(s) in (\"\")"=w96) -> ("States Out"=w94:string)  [unwired: 13 in]
          }
          event "Export": Value Change {
            n36 = event-data() -> ()  [unwired: 1 in, 6 out]
            n37 = call <vilib>:"Add State(s) to Queue__jki_lib_state_machine.vi"("State(s) in Front (\"\")"="Action: Export Calibration", "State(s) in (\"\")"=w100) -> ("States Out"=w101:string)  [unwired: 13 in]
          }
          event "Import": Value Change {
            n38 = event-data() -> ()  [unwired: 1 in, 6 out]
            n39 = call <vilib>:"Add State(s) to Queue__jki_lib_state_machine.vi"("State(s) in Front (\"\")"="Action: Import Calibration", "State(s) in (\"\")"=w105) -> ("States Out"=w106:string)  [unwired: 13 in]
          }
          event "Stop": Value Change {
            n40 = event-data() -> ()  [unwired: 1 in, 6 out]
            n41 = Release Queue(queue=w108, force destroy? (F)=TRUE) -> (error out=w110:errorcluster)  [unwired: 1 in, 2 out]
            n42 = call <vilib>:"Clear Errors.vi"("error in (no error)"=w110) -> ()  [unwired: 5 in, 2 out]
            n43 = call <vilib>:"Add State(s) to Queue__jki_lib_state_machine.vi"("State(s) in Front (\"\")"="Macro: Exit", "State(s) in (\"\")"=w115) -> ("States Out"=w114:string)  [unwired: 13 in]
          }
          event Panel Close? {
            n44 = event-data() -> ()  [unwired: 1 in, 1 out]
            n45 = property on="Stop" class="Bool (strict)"("Val(Sgnl)"=TRUE ("stop")) -> ()  [unwired: 2 in, 2 out]
            n46 = call <vilib>:"Add State(s) to Queue__jki_lib_state_machine.vi"("State(s) in (\"\")"=w121) -> ("States Out"=w120:string)  [unwired: 14 in]
            n47 = event-data("Discard?"=TRUE) -> ()  [unwired: 1 in, 1 out]
          }
        }
      }
      frame "---------- Core ----------" {
        # "Do not put any code in this frame.\n(it is a separator no-op)"
        n48 = call <vilib>:"Add State(s) to Queue__jki_lib_state_machine.vi"("State(s) in (\"\")"=w125) -> ("States Out"=w124:string)  [unwired: 14 in]
      }
      frame Default {
        w135 = 42 items=["No error", "Argument error", "Memory is full", "Out of zone", "End of file", "File already open", "Generic file I/O error", "File not found", "File permission error", "Disk is full", "Duplicate path", "Too many files open", "System feature not enabled", "Resource file not found", "Cannot add resource", "Resource not found", "Image not found", "Image memory error", "Pen does not exist", "Config type invalid", "Config token not found", "Config parse error", "Config memory error", "Bad external code format", "Bad external code offset", "External code not present", "Null window", "Destroy window error", "Null menu", "Print aborted", "Bad print record", "Print driver error", "Windows error during printing", "Memory error during printing", "Print dialog error", "Generic print error", "Invalid device refnum", "Device not found", "Device parameter error", "Device unit error", "Cannot open device", "Device call aborted", "Generic error", "Cancelled by user", "Object ID too low", "Object ID too high", "Object not in heap", "Unknown heap", "Unknown object (invalid DefProc)", "Unknown object (DefProc not in table)", "Message out of range", "Invalid (null) method", "Unknown message", "Manager call not supported", "Bad address", "Network operation in progress", "Network operation timed out", "Connection is busy", "Network attribute not supported", "Network error", "Address in use", "System out of memory", "Connection aborted", "Connection refused", "Not connected", "Already connected", "Connection closed", "Initialization error (interapplication manager)", "Bad occurrence", "Wait on unbound occurrence handler", "Occurrence queue overflow", "Datalog type conflict", "Unused", "Unrecognized type (interapplication manager)", "Memory corrupt", "Failed to make temporary DLL", "Old CIN version", "Drag socket not found", "Failed to load drop-object", "Failed to register OLE object", "Failed to release OLE object", "Format specifier type mismatch", "Unknown format specifier", "Too few format specifiers", "Too many format specifiers", "Scan failed", "Newer CIN version", "Error converting to variant", "Runtime menu error", "Password tampered", "Variant attribute not found", "Incompatible variant data type", "Event data is not available", "Event Store is not present", "Occurrence is not found", "Event Queue is not created", "Event info is not available", "Refnum passed is NULL", "Error retrieving Class GUID", "Error retrieving CoClass GUID", "Error retrieving TypeLib GUID.", "Bad built application magic bytes.", "Specific driver is different from the specific driver associated with the Logical Name.", "There is no session opened to the class driver.", "Max Error", "MAX - Error with config objects", "MAX - Error loading configuration", "MAX - Group not supported"]
        # "Current State"
        # "Do not delete, rename, or modify this frame.\n(this is used to capture unhandled states and typos)"
        # "Handle mistyped state name (developer tool)"
        n49 = Format Into String(format string="Software Exception: Unhandled State \"%s\"." ("message"), error in=w131, w126) -> (resulting string=w134:string, error out=w133:errorcluster)  [unwired: 1 in]
        n50 = call <vilib>:"Error Cluster From Error Code.vi"("show call chain? (False)"=TRUE, "error in (no error)"=w133, "error message (\"\")"=w134, "error code (0)"=w135) -> ("error out"=w132:errorcluster)  [unwired: 5 in]
        n51 = call <vilib>:"Add State(s) to Queue__jki_lib_state_machine.vi"("State(s) in (\"\")"=w130) -> ("States Out"=w129:string)  [unwired: 14 in]
      }
      frame "Initialize Core Data" {
        # "Do not delete, rename, or modify this frame.\n(this is used to determine panel behavior on exit)"
        # "originally closed?"
        # "exe?"
        # "If panel starts closed or is an EXE, then close it when we exit"
        n52 = property class="VI"() -> ("FP.State"=w139:T8)  [unwired: 2 in, 2 out]
        n53 = property class="App"() -> ("App.Kind"=w145:T9)  [unwired: 2 in, 2 out]
        n54 = control-ref of="Current VI Reference"() -> (w140:refnum<vi>)
        n55 = Equal?(x=w139, y=T8."Closed" ("Front Panel Window:State")) -> (x = y?=w137:bool)
        n56 = Equal?(x=w145, y=T9."Run Time System" ("Application:Kind")) -> (x = y?=w143:bool)
        n57 = Or(x=w137, y=w143) -> (x .or. y?=w141:bool)
        n58 = Bundle By Name(cluster=w142, "Core.Current VI Reference"=w140, "Core.Close Panel on Exit?"=w141) -> (w147:T11)
        n59 = call <vilib>:"Add State(s) to Queue__jki_lib_state_machine.vi"("State(s) in (\"\")"=w149) -> ("States Out"=w148:string)  [unwired: 14 in]
      }
      frame "Error Handler" {
        # "Unhandled Error -- Display it"
        # "Handle any errors here.\nYou can also output any states to clean-up after errors occur"
        # "Clear error"
        n60 = call <vilib>:"General Error Handler.vi"("error in (no error)"=w151) -> ()  [unwired: 10 in, 5 out]
        n61 = call <vilib>:"Add State(s) to Queue__jki_lib_state_machine.vi"("State(s) in Front (\"\")"="/* Post Error States", "State(s) in (\"\")"=w155) -> ("States Out"=w154:string)  [unwired: 13 in]
      }
      frame "Exit" {
        # "Do not put any code in this frame.\n(No errors that occur here will be handled.)"
        n62 = call <vilib>:"Add State(s) to Queue__jki_lib_state_machine.vi"("State(s) in (\"\")"=w160) -> ("States Out"=w159:string)  [unwired: 14 in]
      }
      frame "---------- Data ----------" {
        # "Do not put any code in this frame.\n(It is a separator no-op. You can make a copy of this frame to create a new Data frame)"
        n63 = call <vilib>:"Add State(s) to Queue__jki_lib_state_machine.vi"("State(s) in (\"\")"=w164) -> ("States Out"=w163:string)  [unwired: 14 in]
      }
      frame "Data: Initialize" {
        w165 = ""  # Diagnostic type
        w166 = T12 {"Hexapod zscan positions"=[], "Hexapod zscan diagnostic"=[], "Index"=0, "Best Zpos"=0.0}  # Hexapod zscan data
        w167 = cluster{"MaxCounts":dbl, "w0 Y":dbl} {"MaxCounts"=0.0, "w0 Y"=0.0}  # Beam diagnostic cutoffs
        w168 = cluster{"P1":string, "P2":string} {"P1"="", "P2"=""}  # Hexapod positions
        w169 = cluster{"T1":i32, "T2":i32} {"T1"=0, "T2"=0}  # Timer
        w170 = 0  # Alignment attempts
        w171 = 0  # Messages
        w174 = cluster{"X":dbl, "Y":dbl} {"X"=0.01, "Y"=0.02}  # Calibration Angle
        w175 = cluster{"X":dbl, "Y":dbl} {"X"=10.0, "Y"=10.0}  # Accuracy limit
        w176 = 8.0  # Calibration steps
        w177 = T13 {"Centroids.x"=[], "Centroids.y"=[]}  # Centroids
        w178 = cluster{"X":dbl, "Y":dbl} {"X"=0.0, "Y"=0.0}  # Scale Factor
        w179 = cluster{"X":dbl, "Y":dbl} {"X"=0.0, "Y"=0.0}  # Difference
        w180 = T14 {"Current VI Reference"=refnum, "Close Panel on Exit?"=FALSE}  # Core
        # "do not delete - used by framework"
        # "Data names and types of shift register data are defined by this bundle."
        # "Initialize the shift-register data, here.\n(data names are defined by what you wire into the bundle function)"
        n64 = call <vilib>:"Create.vi"("Settings"="Settings") -> ("NetworkConnection out"=w172:refnum<class "NetworkConnection.lvclass">)  [unwired: 9 in, 1 out]
        n65 = Bundle("Core"=w180, "Difference"=w179, "Scale Factor"=w178, "Centroids"=w177, "Calibration Angle"=w174, "Accuracy limit"=w175, "Calibration steps"=w176, "NetworkConnection out"=w172, "Messages"=w171, "Alignment attempts"=w170, "Timer"=w169, "Hexapod positions"=w168, "Beam diagnostic cutoffs"=w167, "Hexapod zscan data"=w166, "Diagnostic type"=w165) -> (w182:T11)  [unwired: 1 in]
        n66 = call <vilib>:"Add State(s) to Queue__jki_lib_state_machine.vi"("State(s) in (\"\")"=w184) -> ("States Out"=w183:string)  [unwired: 14 in]
      }
      frame "Data: Cleanup" {
        # "Cleanup any data and references, here.\n(this is called automatically, by the Macro: Exit)"
        n67 = Unbundle By Name(w188) -> ("Core.Current VI Reference"=w190:refnum<vi>)
        n68 = Close Reference(reference=w190, error in (no error)=w189) -> (error out=w186:errorcluster)
        n69 = Unbundle By Name(w188) -> ("NetworkConnection out"=w187:refnum<class "NetworkConnection.lvclass">)
        n70 = call <vilib>:"Destroy.vi"("error in (no error)"=w186, "NetworkConnection in"=w187) -> ("error out"=w185:errorcluster)  [unwired: 8 in, 1 out]
        n71 = call <vilib>:"Add State(s) to Queue__jki_lib_state_machine.vi"("State(s) in (\"\")"=w192) -> ("States Out"=w191:string)  [unwired: 14 in]
      }
      frame "---------- UI ----------" {
        # "Do not put any code in this frame.\n(It is a separator no-op. You can make a copy of this frame to create a new UI frame)"
        n72 = call <vilib>:"Add State(s) to Queue__jki_lib_state_machine.vi"("State(s) in (\"\")"=w196) -> ("States Out"=w195:string)  [unwired: 14 in]
      }
      frame "UI: Initialize" {
        # "Initialize the User Interface, here.\n(this is called automatically, by the Macro: Init)"
        n73 = call <vilib>:"Add State(s) to Queue__jki_lib_state_machine.vi"("State(s) in (\"\")"=w200) -> ("States Out"=w199:string)  [unwired: 14 in]
      }
      frame "UI: Cursor Set" {
        # "Argument"
        # "Set and Unset Cursor Busy.\n(Usage: \"UI: Cursor Set >> Busy|Idle\")"
        n74 = case shown="\"Idle\", Default" w201 {
          tunnel: w203 -> [w208 w210]
          tunnel: [w207 w209] -> w202
          frame "Idle", Default {
            n75 = call <vilib>:"Unset Busy.vi"("error in (no error)"=w208) -> ("error out"=w207:errorcluster)  [unwired: 10 in]
          }
          frame "Busy" {
            n76 = call <vilib>:"Set Busy.vi"("error in (no error)"=w210) -> ("error out"=w209:errorcluster)  [unwired: 9 in, 1 out]
          }
        }
        n77 = call <vilib>:"Add State(s) to Queue__jki_lib_state_machine.vi"("State(s) in (\"\")"=w206) -> ("States Out"=w205:string)  [unwired: 14 in]
      }
      frame "UI: Front Panel State" {
        # "Argument"
        # "Set Front Panel Open or Closed\n(Usage: \"UI: Front Panel State >> Open|Close\")"
        n78 = Unbundle By Name(w213) -> ("Core.Current VI Reference"=w212:refnum<vi>)
        n79 = case shown="\"Close\", \"Closed\"" w211 {
          tunnel: w215 -> [w223 w238 w249 w262 w275]
          tunnel: [w225 w239 w251 w264 w277] -> w214
          tunnel: w212 -> [w224 w236 w250 w263 w276]
          frame "Open", "Standard", Default {
            w218 = T8."Standard" ("State")
            n80 = property class="VI"(reference=w224, error in=w223) -> (reference out=w221:refnum<vi>, error out=w222:errorcluster, "FP.State"=w220:T8)
            n81 = Not Equal?(x=w220, y=w218) -> (x != y?=w219:bool)
            n82 = case shown="True" w219 {
              tunnel: [w229 w231] -> w225
              tunnel: w222 -> [w228 w231]
              tunnel: w221 -> [w227 _]
              tunnel: w218 -> [w226 _]
              frame True {
                n83 = invoke class="VI" method="FP.Open"(reference=w227, error in=w228, "Activate"=TRUE, "State"=w226) -> (error out=w229:errorcluster)  [unwired: 1 in, 4 out]
              }
              frame False {
              }
            }
          }
          frame "Close", "Closed" {
            n84 = property class="VI"(reference=w236, error in=w238) -> (reference out=w235:refnum<vi>, error out=w237:errorcluster, "FP.State"=w233:T8)
            n85 = Not Equal?(x=w233, y=T8."Closed" ("Front Panel Window:State")) -> (x != y?=w232:bool)
            n86 = case shown="False" w232 {
              tunnel: [w240 w243] -> w239
              tunnel: w237 -> [w240 w242]
              tunnel: w235 -> [_ w241]
              frame False {
              }
              frame True {
                n87 = invoke class="VI" method="FP.Close"(reference=w241, error in=w242) -> (error out=w243:errorcluster)  [unwired: 1 in, 2 out]
              }
            }
          }
          frame "Hidden", "Hide" {
            w244 = T8."Hidden" ("State")
            n88 = property class="VI"(reference=w250, error in=w249) -> (reference out=w247:refnum<vi>, error out=w248:errorcluster, "FP.State"=w246:T8)
            n89 = Not Equal?(x=w246, y=w244) -> (x != y?=w245:bool)
            n90 = case shown="True" w245 {
              tunnel: [w255 w256] -> w251
              tunnel: w248 -> [w254 w256]
              tunnel: w247 -> [w253 _]
              tunnel: w244 -> [w252 _]
              frame True {
                n91 = invoke class="VI" method="FP.Open"(reference=w253, error in=w254, "State"=w252) -> (error out=w255:errorcluster)  [unwired: 2 in, 4 out]
              }
              frame False {
              }
            }
          }
          frame "Minimize", "Minimized" {
            w257 = T8."Minimized" ("State")
            n92 = property class="VI"(reference=w263, error in=w262) -> (reference out=w260:refnum<vi>, error out=w261:errorcluster, "FP.State"=w259:T8)
            n93 = Not Equal?(x=w259, y=w257) -> (x != y?=w258:bool)
            n94 = case shown="True" w258 {
              tunnel: [w268 w269] -> w264
              tunnel: w261 -> [w267 w269]
              tunnel: w260 -> [w266 _]
              tunnel: w257 -> [w265 _]
              frame True {
                n95 = invoke class="VI" method="FP.Open"(reference=w266, error in=w267, "State"=w265) -> (error out=w268:errorcluster)  [unwired: 2 in, 4 out]
              }
              frame False {
              }
            }
          }
          frame "Maximize", "Maximized" {
            w270 = T8."Maximized" ("State")
            n96 = property class="VI"(reference=w276, error in=w275) -> (reference out=w273:refnum<vi>, error out=w274:errorcluster, "FP.State"=w272:T8)
            n97 = Not Equal?(x=w272, y=w270) -> (x != y?=w271:bool)
            n98 = case shown="True" w271 {
              tunnel: [w281 w282] -> w277
              tunnel: w274 -> [w280 w282]
              tunnel: w273 -> [w279 _]
              tunnel: w270 -> [w278 _]
              frame True {
                n99 = invoke class="VI" method="FP.Open"(reference=w279, error in=w280, "State"=w278) -> (error out=w281:errorcluster)  [unwired: 2 in, 4 out]
              }
              frame False {
              }
            }
          }
        }
        n100 = call <vilib>:"Add State(s) to Queue__jki_lib_state_machine.vi"("State(s) in (\"\")"=w217) -> ("States Out"=w216:string)  [unwired: 14 in]
      }
      frame "---------- Macro ----------" {
        # "Do not put any code in this frame.\n(It is a separator no-op. You can make a copy of this frame to create a new Macro frame)"
        n101 = call <vilib>:"Add State(s) to Queue__jki_lib_state_machine.vi"("State(s) in (\"\")"=w286) -> ("States Out"=w285:string)  [unwired: 14 in]
      }
      frame "Macro: Initialize" {
        # "Initialization Macro\n(This is called once, when the VI starts)"
        n102 = call <vilib>:"Add State(s) to Queue__jki_lib_state_machine.vi"("State(s) in Front (\"\")"="Data: Initialize\nInitialize Core Data\nUI: Initialize\nUI: Front Panel State >> Open", "State(s) in (\"\")"=w291) -> ("States Out"=w290:string)  [unwired: 13 in]
      }
      frame "Macro: Calibrate" {
        w293 = dbl[] []
        # "Create the state list for calibration"
        # "Empty the array"
        n103 = Unbundle By Name(w294) -> ("Calibration steps"=w295:dbl)
        n104 = call <vilib>:"Add State(s) to Queue__jki_lib_state_machine.vi"("State(s) in Front (\"\")"="Action: Get Centroid>> Calibrate", "State(s) in (\"\")"=w301) -> ("States Out"=w300:string)  [unwired: 13 in]
        n105 = Subtract(x=w295, y=1.0) -> (x-y=w298:dbl)
        n106 = for {
          N: w298 -> [_]
          shift-right: [w305] -> w296
          shift-left: w300 -> [w307]
          n107 = call <vilib>:"Add State(s) to Queue__jki_lib_state_machine.vi"("State(s) in (\"\")"=w307, "State(s) at Back (\"\")"="Action: Move>> Calibrate\nAction: Get Centroid>> Calibrate") -> ("States Out"=w305:string)  [unwired: 13 in]
        }
        n108 = call <vilib>:"Add State(s) to Queue__jki_lib_state_machine.vi"("State(s) in (\"\")"=w296, "State(s) at Back (\"\")"="Action: Calibrate" ("State(s) in Front (\"\")")) -> ("States Out"=w304:string)  [unwired: 13 in]
        n109 = Bundle By Name(cluster=w294, "Centroids.Centroids.x"=w293, "Centroids.Centroids.y"=w293) -> (w292:T11)
      }
      frame "Macro: Hexapod Zpos Scan" {
        n110 = local read "zpos::2"() -> (w321:dbl)
        n111 = case shown="\"w0 Y\"" "Diagnostic type" {
          tunnel: ["maxcounts" "w0y"] -> w308
          frame "Max counts", Default {
          }
          frame "w0 Y" {
          }
        }
        n112 = Divide(x="zpos scan range", y=2) -> (x/y=w320:dbl)
        n113 = Divide(x="zpos scan range", y="zpos scan increment") -> (x/y=w327:dbl)
        n114 = Subtract(x=w321, y=w320) -> (x-y=w319:dbl)
        n115 = Increment(x=w327) -> (x+1=w315:dbl)
        n116 = for {
          N: w315 -> [_]
          tunnel: [w335] -> w326 mode=indexing
          i -> [w335]
        }
        n117 = Multiply(x=w326, y="zpos scan increment") -> (x*y=w324:dbl[])
        n118 = for {
          N: w315 -> [_]
          shift-right: [w332] -> w312
          shift-left: w313 -> [w334]
          n119 = call <vilib>:"Add State(s) to Queue__jki_lib_state_machine.vi"("State(s) in Front (\"\")"="Action: Move>> Zpos Scan \nAction: Get Beam Diagnostic>> Zpos Scan", "State(s) in (\"\")"=w334) -> ("States Out"=w332:string)  [unwired: 13 in]
        }
        n120 = Add(x=w319, y=w324) -> (x+y=w318:dbl[])
        n121 = Bundle By Name(cluster=w317, "Hexapod zscan data.Hexapod zscan positions"=w318, "Hexapod zscan data.Index"=0, "Hexapod zscan data.Hexapod zscan diagnostic"=dbl[] [], "Diagnostic type"=w308) -> (w316:T11)
        n122 = call <vilib>:"Add State(s) to Queue__jki_lib_state_machine.vi"("State(s) in (\"\")"=w312, "State(s) at Back (\"\")"="Action: Find Best Zpos") -> ("States Out"=w329:string)  [unwired: 13 in]
      }
      frame "Macro: Alignment" {
        # "Create initial state list for alignment"
        n123 = Tick Count (ms)() -> (millisecond timer value=w338:u32)
        n124 = Bundle By Name(cluster=w336, "Timer.T1"=w338) -> (w337:T11)
        n125 = call <vilib>:"Add State(s) to Queue__jki_lib_state_machine.vi"("State(s) in Front (\"\")"="Update: Alignment Constants\nAction: Get Centroid>> Align", "State(s) in (\"\")"=w340) -> ("States Out"=w342:string)  [unwired: 13 in]
      }
      frame "Macro: Exit" {
        # "Exit Macro\n(This is called once, when the VI exits)"
        n126 = disable-structure shown="Enabled" {
          disable-tunnel: w349 -> [w354 _]
          disable-tunnel: [w353 FALSE ("Close Panel on Exit?")] -> w344
          frame Disabled {
            n127 = Unbundle By Name(w354) -> ("Core.Close Panel on Exit?"=w353:bool)
          }
          frame Enabled {
          }
        }
        n128 = Select(t="UI: Front Panel State >> Close", s=w344, f="") -> (s? t:f=w347:string)
        n129 = call <vilib>:"Add State(s) to Queue__jki_lib_state_machine.vi"("State(s) in (\"\")"=w347, "State(s) at Back (\"\")"="Data: Cleanup\nExit") -> ("States Out"=w345:string)  [unwired: 13 in]
        n130 = call <vilib>:"Add State(s) to Queue__jki_lib_state_machine.vi"("State(s) in Front (\"\")"=w345, "State(s) in (\"\")"=w352) -> ("States Out"=w351:string)  [unwired: 13 in]
      }
      frame "---------- Update ----------" {
        # "Do not put any code in this frame.\n(It is a separator no-op. You can make a copy of this frame to create a new Macro frame)"
        n131 = call <vilib>:"Add State(s) to Queue__jki_lib_state_machine.vi"("State(s) in (\"\")"=w359) -> ("States Out"=w358:string)  [unwired: 14 in]
      }
      frame "Update: Calibration Constants" {
        n132 = Bundle By Name(cluster=w363, "Calibration steps"="Calibration steps", "Calibration Angle"="Calibration Angle", "Alignment attempts"=0) -> (w362:T11)
        n133 = call <vilib>:"Add State(s) to Queue__jki_lib_state_machine.vi"("State(s) in (\"\")"=w365) -> ("States Out"=w367:string)  [unwired: 14 in]
      }
      frame "Update: Alignment Constants" {
        n134 = Bundle By Name(cluster=w372, "Accuracy limit"="Accuracy limit", "Alignment attempts"=0) -> (w371:T11)
        n135 = call <vilib>:"Add State(s) to Queue__jki_lib_state_machine.vi"("State(s) in (\"\")"=w373) -> ("States Out"=w374:string)  [unwired: 14 in]
      }
      frame "---------- Action ----------" {
        # "Do not put any code in this frame.\n(It is a separator no-op. You can make a copy of this frame to create a new Macro frame)"
        n136 = call <vilib>:"Add State(s) to Queue__jki_lib_state_machine.vi"("State(s) in (\"\")"=w378) -> ("States Out"=w377:string)  [unwired: 14 in]
      }
      frame "Action: Get Centroid" {
        n137 = case shown="\"Align\", Default" w388 {
          tunnel: w387 -> [w394 w417]
          tunnel: "centroidy::1" -> [w396 w403]
          tunnel: "centroidx::1" -> [w395 w402]
          tunnel: [w393 w413] -> w386
          tunnel: "Target.X::1" -> [_ w416]
          tunnel: "Target.Y::1" -> [_ w415]
          tunnel: ["" w414] -> w385
          tunnel: w379 -> [w391 w401]
          tunnel: [w391 w401] -> w380
          frame "Calibrate" {
            # "Reads centroid position and adds them to array for calibration calculation"
            n138 = Unbundle By Name(w394) -> ("Centroids.Centroids.x"=w397:dbl[], "Centroids.Centroids.y"=w398:dbl[])
            n139 = Build Array (concatenate)(w397, w395) -> (w399:dbl[])
            n140 = Build Array (concatenate)(w398, w396) -> (w400:dbl[])
            n141 = Bundle By Name(cluster=w394, "Centroids.Centroids.x"=w399, "Centroids.Centroids.y"=w400) -> (w393:T11)
          }
          frame "Align", Default {
            # "After movement, check if difference between centroid and target is within tolerance. If it is within tolerance, end alignment. If it isn't within tolerance, move hexapod again."
            n142 = Unbundle By Name(w417) -> ("Accuracy limit.X"=w412:dbl, "Accuracy limit.Y"=w410:dbl)
            n143 = Subtract(x=w416, y=w402) -> (x-y=w419:dbl)
            n144 = Subtract(x=w415, y=w403) -> (x-y=w418:dbl)
            n145 = Bundle By Name(cluster=w417, "Difference.X"=w419, "Difference.Y"=w418) -> (w413:T11)
            n146 = Absolute Value(x=w419) -> (abs(x)=w411:dbl)
            n147 = Absolute Value(x=w418) -> (abs(x)=w409:dbl)
            n148 = Greater?(x=w412, y=w411) -> (0:w405:bool)
            n149 = Greater?(x=w410, y=w409) -> (0:w406:bool)
            n150 = And(x=w405, y=w406) -> (x .and. y?=w404:bool)
            n151 = Select(t=" Action: Send Response ", s=w404, f="Action: Move>> Align\nAction: Get Centroid>> Align") -> (s? t:f=w414:string)
            n152 = case shown="True" w404 {
              tunnel: w403 -> [_ w422]
              tunnel: w402 -> [_ w420]
              frame False {
              }
              frame True {
                n153 = Bundle("centroidx::1"=w420, "centroidy::1"=w422) -> (→"Waveform Chart":cluster{"centroidx::1":dbl, "centroidy::1":dbl})  [unwired: 1 in]
              }
            }
          }
        }
        n154 = call <vilib>:"Add State(s) to Queue__jki_lib_state_machine.vi"("State(s) in Front (\"\")"=w385, "State(s) in (\"\")"=w390) -> ("States Out"=w389:string)  [unwired: 13 in]
      }
      frame "Action: Move" {
        # "send movement command to hexapod\nand wait for slow response"
        n155 = case shown="\"Calibrate\"" w447 {
          tunnel: w446 -> [w477 w491 w516 w526]
          tunnel: "xpos::2" -> [w488 w506 w525 w533]
          tunnel: [w488 w506 w525 w533] -> w437
          tunnel: "ypos::2" -> [w487 w505 w524 w532]
          tunnel: [w487 w505 w524 w532] -> w435
          tunnel: "zpos::2" -> [w479 w504 _ _]
          tunnel: [w479 w504 w518 w528] -> w433
          tunnel: "uangle::2" -> [w480 w497 w523 w531]
          tunnel: [w480 w497 w523 w531] -> w431
          tunnel: "wangle::2" -> [w485 w503 w521 w529]
          tunnel: [w484 w501 w521 w529] -> w429
          tunnel: "vangle::2" -> [w482 w500 w522 w530]
          tunnel: [w481 w498 w522 w530] -> w427
          tunnel: w426 -> [w478 w493 w517 w527]
          tunnel: [w478 w490 w517 w527] -> w425
          tunnel: [w477 w489 w516 w526] -> w424
          frame "Calibrate" {
            # "Calibration movement"
            n156 = Unbundle By Name(w477) -> ("Calibration Angle.Y"=w483:dbl, "Calibration Angle.X"=w486:dbl)
            n157 = Add(x=w482, y=w483) -> (x+y=w481:dbl)
            n158 = Add(x=w486, y=w485) -> (x+y=w484:dbl)
          }
          frame "Align", Default {
            # "Correction movement, scaled by a factor"
            n159 = Unbundle By Name(w491) -> ("Alignment attempts"=w494:i32)
            n160 = Unbundle By Name(w491) -> ("Difference.Y"=w513:dbl, "Scale Factor.Y"=w512:dbl, "Difference.X"=w511:dbl, "Scale Factor.X"=w510:dbl)
            n161 = Multiply(x=w511, y=w510) -> (x*y=w508:dbl)
            n162 = Multiply(x=w513, y=w512) -> (x*y=w509:dbl)
            n163 = Increment(x=w494) -> (x+1=w496:i32)
            "Alignment attempts" <- w496
            n164 = Multiply(x="Buffer", y=w508) -> (x*y=w502:dbl)
            n165 = Multiply(x=w509, y="Buffer") -> (x*y=w499:dbl)
            n166 = Add(x=w499, y=w500) -> (x+y=w498:dbl)
            n167 = Add(x=w502, y=w503) -> (x+y=w501:dbl)
            n168 = Greater?(x=w496, y=10) -> (0:w495:bool)
            n169 = Bundle By Name(cluster=w491, "Alignment attempts"=w496) -> (w489:T11)
            n170 = case shown="True" w495 {
              tunnel: [w514 ""] -> w490
              tunnel: w493 -> [w514 _]
              frame False {
              }
              frame True {
              }
            }
          }
          frame "Zpos Scan" {
            n171 = Unbundle By Name(w516) -> ("Hexapod zscan data.Index"=w520:i32, "Hexapod zscan data.Hexapod zscan positions"=w519:dbl[])
            n172 = Index Array(array=w519, index=w520) -> (element=w518:dbl)
          }
          frame "Best Zpos" {
            n173 = Unbundle By Name(w526) -> ("Hexapod zscan data.Best Zpos"=w528:dbl)
          }
        }
        n174 = call <userlib>:"Tick Count (ms)__ogtk.vi"("error in (no error)"=w445) -> ("error out"=w441:errorcluster, "millisecond timer value"=w443:u32)  [unwired: 9 in]
        n175 = disable-structure "Diagram Disable Structure" shown="Enabled" {
          disable-tunnel: w437 -> [w464 _]
          disable-tunnel: w435 -> [w463 _]
          disable-tunnel: w433 -> [w462 _]
          disable-tunnel: w431 -> [w461 _]
          disable-tunnel: w427 -> [w460 w472]
          disable-tunnel: w429 -> [w459 w473]
          disable-tunnel: "GUIdevice 2" -> [w451 w469]
          disable-tunnel: w441 -> [w453 w476]
          disable-tunnel: [w450 w474] -> w440
          frame Enabled {
            # "create command"
            # "turn into proper formatting"
            # "convert to string"
            # "create hexapod state array"
            # "Full xyzuvw command structure"
            n176 = Build Array(w464, w463, w462, w461, w460, w459) -> (w458:dbl[])
            n177 = Number To Fractional String(number=w458) -> (F-format string=w457:string[])  [unwired: 3 in]
            n178 = call <userlib>:"1D Array to String__ogtk.vi"("delimiter (Tab)"="," ("string"), "Array of Strings"=w457) -> ("delimited string"=w454:string)  [unwired: 9 in]
            n179 = Concatenate Strings("setxyzuvw>>" ("command in"), w454) -> (w452:string)
            n180 = call "send udp and wait for slow response.vi"("error in"=w453, "command in"=w452, "Device"=w451) -> ("error out"=w450:errorcluster, "slow response"=→"slow response":string)  [unwired: 5 in, 2 out]
          }
          frame Disabled {
            # "separate w and v angle commands"
            n181 = Number To Fractional String(number=w473) -> (F-format string=w470:string)  [unwired: 3 in]
            n182 = Number To Fractional String(number=w472) -> (F-format string=w467:string)  [unwired: 3 in]
            n183 = Concatenate Strings("setwangle >>", w470) -> (w468:string)
            n184 = Concatenate Strings("setvangle>>", w467) -> (w465:string)
            n185 = call "send udp and wait for slow response.vi"("error in"=w476, "command in"=w468, "Device"=w469) -> ("error out"=w475:errorcluster)  [unwired: 5 in, 3 out]
            n186 = call "send udp and wait for slow response.vi"("error in"=w475, "command in"=w465, "Device"=w469) -> ("error out"=w474:errorcluster)  [unwired: 5 in, 3 out]
          }
        }
        n187 = call <userlib>:"Tick Count (ms)__ogtk.vi"("error in (no error)"=w440) -> ("error out"=w439:errorcluster, "millisecond timer value"=w444:u32)  [unwired: 9 in]
        n188 = Subtract(x=w444, y=w443) -> (x-y=→"Waveform Chart 2" →"Movement time":u32)
        n189 = call <vilib>:"Add State(s) to Queue__jki_lib_state_machine.vi"("State(s) in (\"\")"=w425) -> ("States Out"=w448:string)  [unwired: 14 in]
      }
      frame "Action: Calibrate" {
        # "Same as below but for x data"
        # "linear regression fit of data"
        # "cluster of best fit data"
        # "cluster of actual data"
        # "Create array of calibration steps"
        n190 = Unbundle By Name(w554) -> ("Calibration steps"=w547:dbl, "Calibration Angle.X"=w553:dbl, "Centroids.Centroids.x"=w537:dbl[], "Calibration Angle.Y"=w536:dbl, "Centroids.Centroids.y"=w546:dbl[])
        n191 = for {
          N: w547 -> [_]
          tunnel: [w559] -> w552 mode=indexing
          i -> [w559]
        }
        n192 = Multiply(x=w552, y=w536) -> (x*y=w550:dbl[])
        n193 = Multiply(x=w553, y=w552) -> (x*y=w551:dbl[])
        n194 = Bundle("Centroids.x"=w537, w551) -> (w542:cluster{"Centroids.x":dbl[], dbl[]})  [unwired: 1 in]
        n195 = call <vilib>:"Linear Fit.vi"("Y"=w551, "X"=w537) -> ("Best Linear Fit"=w534:dbl[], "slope"=w549:dbl, "residue"=→"X error":dbl)  [unwired: 9 in, 2 out]
        "X slope" <- w549
        n196 = Bundle("Centroids.y"=w546, w550) -> (w544:cluster{"Centroids.y":dbl[], dbl[]})  [unwired: 1 in]
        n197 = call <vilib>:"Linear Fit.vi"("Y"=w550, "X"=w546) -> ("Best Linear Fit"=w535:dbl[], "slope"=w548:dbl, "residue"=→"Y error":dbl)  [unwired: 9 in, 2 out]
        "Y slope" <- w548
        n198 = Bundle("Centroids.x"=w537, "Best Linear Fit"=w534) -> (w541:T15)  [unwired: 1 in]
        n199 = Bundle("Centroids.y"=w546, "Best Linear Fit"=w535) -> (w545:T16)  [unwired: 1 in]
        n200 = Build Array(w542, w541) -> (→"X Graph":T2)
        n201 = Build Array(w544, w545) -> (→"Y Graph":T3)
        n202 = Bundle By Name(cluster=w554, "Scale Factor.X"=w549, "Scale Factor.Y"=w548) -> (w555:T11)
        n203 = call <vilib>:"Add State(s) to Queue__jki_lib_state_machine.vi"("State(s) in (\"\")"=w558) -> ("States Out"=w557:string)  [unwired: 14 in]
      }
      frame "Action: Export Calibration" {
        n204 = Unbundle By Name(w564) -> ("Scale Factor"=w563:cluster{"X":dbl, "Y":dbl})
        n205 = call <userlib>:"MGI Write Anything.vi"("Error In"=w561, "Section Name (Name of \"Anything\")"="Calibration", "Anything"=w563) -> ("Error Out"=w560:errorcluster)  [unwired: 6 in, 2 out]
        n206 = call <vilib>:"Add State(s) to Queue__jki_lib_state_machine.vi"("State(s) in (\"\")"=w566) -> ("States Out"=w565:string)  [unwired: 14 in]
      }
      frame "Action: Import Calibration" {
        n207 = Unbundle By Name(w572) -> ("Scale Factor"=w571:cluster{"X":dbl, "Y":dbl})
        n208 = call <userlib>:"MGI Read Anything.vi"("Type of Anything"=w571, "Error In"=w568, "Section Name (Name of \"Type of Anything\")"="Calibration") -> ("Error Out"=w574:errorcluster, "Anything"=w573:variant)  [unwired: 5 in, 2 out]
        n209 = Variant To Data(error in=w574, type=w571, Variant=w573) -> (data=w570:cluster{"X":dbl, "Y":dbl}, error out=w567:errorcluster)
        n210 = Bundle By Name(cluster=w572, "Scale Factor"=w570) -> (w575:T11)
        n211 = call <vilib>:"Add State(s) to Queue__jki_lib_state_machine.vi"("State(s) in (\"\")"=w577) -> ("States Out"=w576:string)  [unwired: 14 in]
      }
      frame "Action: Get Beam Diagnostic" {
        n212 = Unbundle By Name(w579) -> ("Diagnostic type"=w578:string)
        n213 = case shown="\"maxcounts\", Default" w578 {
          tunnel: ["MaxCounts::1" "2ndmomW0y::1"] -> w585
          tunnel: ["Max counts cutoff" "w0 Y Cutoff"] -> w580
          frame "maxcounts", Default {
          }
          frame "w0y" {
          }
        }
        n214 = case shown="\"Check Quality\", Default" w586 {
          tunnel: w579 -> [w598 w609]
          tunnel: w585 -> [w602 w614]
          tunnel: [w599 ""] -> w584
          tunnel: [w598 w613] -> w583
          tunnel: w582 -> [w595 w607]
          tunnel: [w595 w607] -> w581
          tunnel: w580 -> [w593 _]
          frame "Check Quality", Default {
            n215 = Greater?(x=w602, y=w593) -> (0:w601:bool)
            n216 = case shown="True" "Disable pointing correction" {
              tunnel: ["Macro: Alignment" ""] -> w594
              frame False {
              }
              frame True {
              }
            }
            n217 = case shown="False" "Disable Zpos Scan" {
              tunnel: ["Macro: Hexapod Zpos Scan" w606] -> w600
              tunnel: w594 -> [_ w606]
              frame False {
              }
              frame True {
              }
            }
            n218 = Select(t=w600, s=w601, f=w594) -> (s? t:f=w599:string)
          }
          frame "Zpos Scan" {
            n219 = Unbundle By Name(w609) -> ("Hexapod zscan data.Hexapod zscan diagnostic"=w615:dbl[], "Hexapod zscan data.Index"=w611:i32)
            n220 = Build Array (concatenate)(w615, w614) -> (w612:dbl[])
            n221 = Increment(x=w611) -> (x+1=w610:i32)
            n222 = Bundle By Name(cluster=w609, "Hexapod zscan data.Hexapod zscan diagnostic"=w612, "Hexapod zscan data.Index"=w610) -> (w613:T11)
          }
        }
        n223 = call <vilib>:"Add State(s) to Queue__jki_lib_state_machine.vi"("State(s) in Front (\"\")"=w584, "State(s) in (\"\")"=w588) -> ("States Out"=w587:string)  [unwired: 13 in]
      }
      frame "Action: Find Best Zpos" {
        n224 = Unbundle By Name(w624) -> ("Hexapod zscan data.Hexapod zscan positions"=w621:dbl[], "Hexapod zscan data.Hexapod zscan diagnostic"=w622:dbl[], "Diagnostic type"=w616:string)
        n225 = case shown="\"Max counts\", Default" w616 {
          tunnel: w622 -> [w630 w633]
          tunnel: [w629 w632] -> w619
          tunnel: [w628 w631] -> w618
          frame "Max counts", Default {
            n226 = Array Max & Min(array=w630) -> (max value=w628:dbl, max index (indices)=w629:i32)  [unwired: 2 out]
          }
          frame "w0 Y" {
            n227 = Array Max & Min(array=w633) -> (min value=w631:dbl, min index (indices)=w632:i32)  [unwired: 2 out]
          }
        }
        "Zpos and w0 Y 2" <- w618
        n228 = Index Array(array=w621, index=w619) -> (element=w617:dbl)
        "Zpos and w0 Y" <- w617
        n229 = Bundle By Name(cluster=w624, "Hexapod zscan data.Best Zpos"=w617) -> (w623:T11)
        n230 = call <vilib>:"Add State(s) to Queue__jki_lib_state_machine.vi"("State(s) in Front (\"\")"="Action: Move>> Best Zpos\nMacro: Alignment", "State(s) in (\"\")"=w627) -> ("States Out"=w626:string)  [unwired: 13 in]
      }
      frame "Action: Send Response" {
        n231 = Unbundle By Name(w644) -> ("NetworkConnection out"=w647:refnum<class "NetworkConnection.lvclass">, "Messages"=w641:i32, "Timer.T1"=w636:i32, "Alignment attempts"=→"Waveform Chart 4":i32)
        "Message count" <- w641
        n232 = Bundle By Name(cluster="Message To Send", "Msg Id"=w641) -> (w642:T4)
        n233 = Increment(x=w641) -> (x+1=w640:i32)
        n234 = call <vilib>:"WriteMessage.vi"("Timeout(ms)"=500, "error in (no error)"=w648, "Message"=w642, "NetworkConnection in"=w647) -> ("error out"=w639:errorcluster, "NetworkConnection out"=w646:refnum<class "NetworkConnection.lvclass">)  [unwired: 4 in, 2 out]
        n235 = call <userlib>:"Tick Count (ms)__ogtk.vi"("error in (no error)"=w639) -> ("error out"=w638:errorcluster, "millisecond timer value"=w637:u32)  [unwired: 9 in]
        n236 = Subtract(x=w637, y=w636) -> (x-y=→"Alignment time" →"Waveform Chart 3":u32)
        n237 = Bundle By Name(cluster=w644, "NetworkConnection out"=w646, "Messages"=w640, "Timer.T2"=w637) -> (w645:T11)
        n238 = call <vilib>:"Add State(s) to Queue__jki_lib_state_machine.vi"("State(s) in (\"\")"=w651) -> ("States Out"=w650:string)  [unwired: 14 in]
      }
    }
  }
